vi "UI_page1.vi"(10 "传递队列输入":refnum<queue>, 11 "notifier":refnum<notifier>) -> ()   [LabVIEW 2012]
uses:
  <vilib>/GPower/VIRegister/Library/Convert/ToStr.vi
  <vilib>/GPower/VIRegister/Library/Convert/ToSGLArry.vi
  <vilib>/GPower/VIRegister/Library/Convert/ToI32.vi
  <vilib>/GPower/VIRegister/Library/SubVIs/FindRegisterData.vi
  <vilib>/GPower/VIRegister/Library/SubVIs/ReadSub.vi
  <vilib>/GPower/VIRegister/Library/SubVIs/WriteSub.vi
  <vilib>/GPower/VIRegister/Library/QManager/GetRegisterData.vi
  <vilib>/GPower/Error/Library/SetError.vi
  <vilib>/GPower/Error/Library/FilterCodes.vi
  <vilib>/GPower/Error/Library/Filter/FilterMulti.vi
  <vilib>/GPower/VIRegister/Library/QManager/QManagerAction.vi
  <vilib>/GPower/Error/Library/ErrorType.vi
  <vilib>/GPower/Error/Library/SplitAppended.vi
  <vilib>/GPower/Error/Library/SubVIs/ExplanationToError.vi
  <vilib>/GPower/VIRegister/Library/QManager/GetQName.vi
  <vilib>/GPower/VIRegister/Library/QManager/StartQManager.vi
  <vilib>/Utility/error.llb/Trim Whitespace.vi
  <vilib>/dlg_ctls.llb/Space Constant.vi
  <vilib>/Utility/error.llb/Error Code Database.vi
  <vilib>/GPower/Error/Library/SubVIs/SetStatus.vi
  <vilib>/GPower/Error/Library/AppendErrors.vi
  <vilib>/GPower/Error/Library/Append/AppendSingle.vi
  <vilib>/GPower/VIRegister/VIRegister.lvlib
  <vilib>/measure/NI_MABase.lvlib
panel:
  in  "选项卡控件":enum32{"光纤惯组数据设置", "主份1553B数据", "备份1553B数据"}(tab)
  in  "加表频率":dbl
  in  "加表幅值":dbl
  in  "陀螺频率":dbl
  in  "陀螺幅值":dbl
  in  "地检按钮":bool
  out "中断计数":i32
  out "模拟量显示区":string
  out "备份自检状态及船舱标志":string
  out "主份自检状态及船舱标志":string
  out "接收数据统计区域":string
  in  "备份加计3断电":bool
  in  "备份加计3加电":bool
  in  "备份陀螺3断电":bool
  in  "备份陀螺3加电":bool
  in  "备份温控关闭":bool
  in  "备份加计2断电":bool
  in  "备份加计1断电":bool
  in  "备份加计2加电":bool
  in  "备份加计1加电":bool
  in  "备份陀螺2断电":bool
  in  "备份陀螺1断电":bool
  in  "备份陀螺2加电":bool
  in  "备份陀螺1加电":bool
  in  "备份温控开启":bool
  in  "备份复位":bool
  in  "主份加计3断电":bool
  in  "主份加计3加电":bool
  in  "主份陀螺3断电":bool
  in  "主份陀螺3加电":bool
  in  "主份温控关闭":bool
  in  "主份加计2断电":bool
  in  "主份加计1断电":bool
  in  "主份加计2加电":bool
  in  "主份加计1加电":bool
  in  "主份陀螺2断电":bool
  in  "主份陀螺1断电":bool
  in  "主份陀螺2加电":bool
  in  "主份陀螺1加电":bool
  in  "主份温控开启":bool
  in  "主份复位":bool
  in  "备份复位远程终端":bool
  in  "备份取消发送器关闭":bool
  in  "备份发送器关闭":bool
  in  "备份发送上一状态字":bool
  in  "主份复位远程终端":bool
  in  "主份取消发送器关闭":bool
  in  "主份发送器关闭":bool
  in  "主份发送上一状态字":bool
  in  "备份RT地址选择":enum32{"RT31", "RT21", "RT9"}(radio)
  in  "主份RT地址选择":enum32{"RT31", "RT21", "RT9"}(radio)
  in  "备份通道选择":enum32{"通道A", "通道B"}(radio)
  in  "主份通道选择":enum32{"通道A", "通道B"}(radio)
  in  "备份自定义周期":dbl caption="ms"
  in  "备份周期设置":enum32{"160ms", "自定义", "480ms"}(radio)
  in  "主份自定义周期":dbl caption="ms"
  in  "主份周期设置":enum32{"160ms", "自定义", "480ms"}(radio)
  in  "设置存储信息":bool
  in  "备份存储":bool
  in  "主份存储":bool
  out "波形图表 12":dbl(graph)
  out "波形图表 11":dbl(graph)
  out "波形图表 10":dbl(graph)
  out "波形图表 9":dbl(graph)
  out "波形图表 8":dbl(graph)
  out "波形图表 7":dbl(graph)
  out "波形图表 6":dbl(graph)
  out "波形图表 5":dbl(graph)
  out "波形图表 4":dbl(graph)
  out "波形图表 3":dbl(graph)
  out "波形图表 2":dbl(graph)
  out "波形图表":dbl(graph)
  # "主份模式指令"
  # "测量存储区"
  # "备份模式指令"
  # "主份指令"
  # "备份指令"
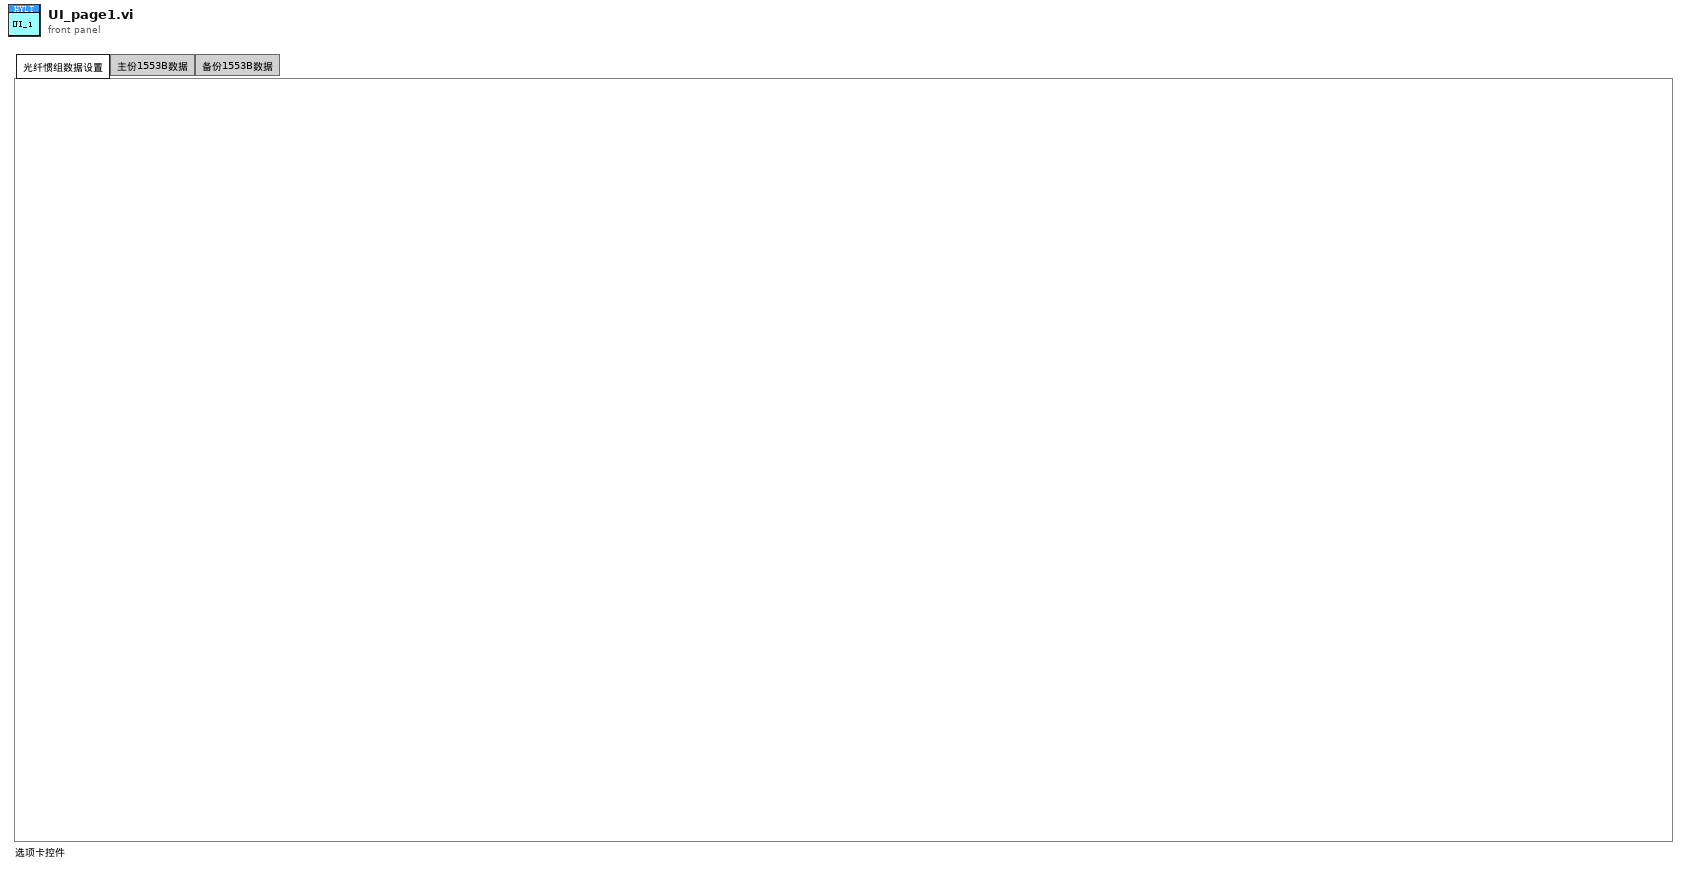
[diagram p1: front panel]
types:
  T1 = cluster{"主份通道选择":enum32{"通道A", "通道B"}, "备份通道选择":enum32{"通道A", "通道B"}}
  T2 = enum32{"invalid app kind", "Development System", "Run Time System", "Student Edition", "Embedded LabVIEW", "Evaluation", "Custom"}
  T3 = enum32{"Invalid", "Standard", "Closed", "Hidden", "Minimized", "Maximized"}
  T4 = cluster{"Core":cluster{"Current VI Reference":refnum<vi>, "Close Panel on Exit?":bool}, "传递队列输入":refnum<queue>, "信息帧":cluster{" 数据帧名称":string, " 数据":string, "备用操作符":bool, "起始地址":i32, "读写标志":i32, "长度":i32}, "主份控制指令":u16, "备份控制指令":u16}
  T5 = cluster{" 数据帧名称":string, " 数据":string, "备用操作符":bool, "起始地址":i32, "读写标志":i32, "长度":i32}
  T6 = cluster{"Current VI Reference":refnum<vi>, "Close Panel on Exit?":bool}
  T7 = cluster{"G1陀螺脉冲数":u32, "G2陀螺脉冲数":u32, "G3陀螺脉冲数":u32, "A1加速度计脉冲数":u32, "A2加速度计脉冲数":u32, "A3加速度计脉冲数":u32, "G1陀螺自检状态":u8, "G1陀螺光路温度":u8, "G2陀螺自检状态":u8, "G2陀螺光路温度":u8, "G3陀螺自检状态":u8, "G3陀螺光路温度":u8, "A1自检状态":u8, "A1幅值":u8, "A2自检状态":u8, "A2幅值":u8, "A3自检状态":u8, "A3幅值":u8, "IF1电路温度":u8, "IF2电路温度":u8, "IF3电路温度":u8, "温控自检字":u8, "加速度计温度测量字1":u32, "加速度计温度测量字2":u32, "LTU状态":u8, "帧计数":u8}
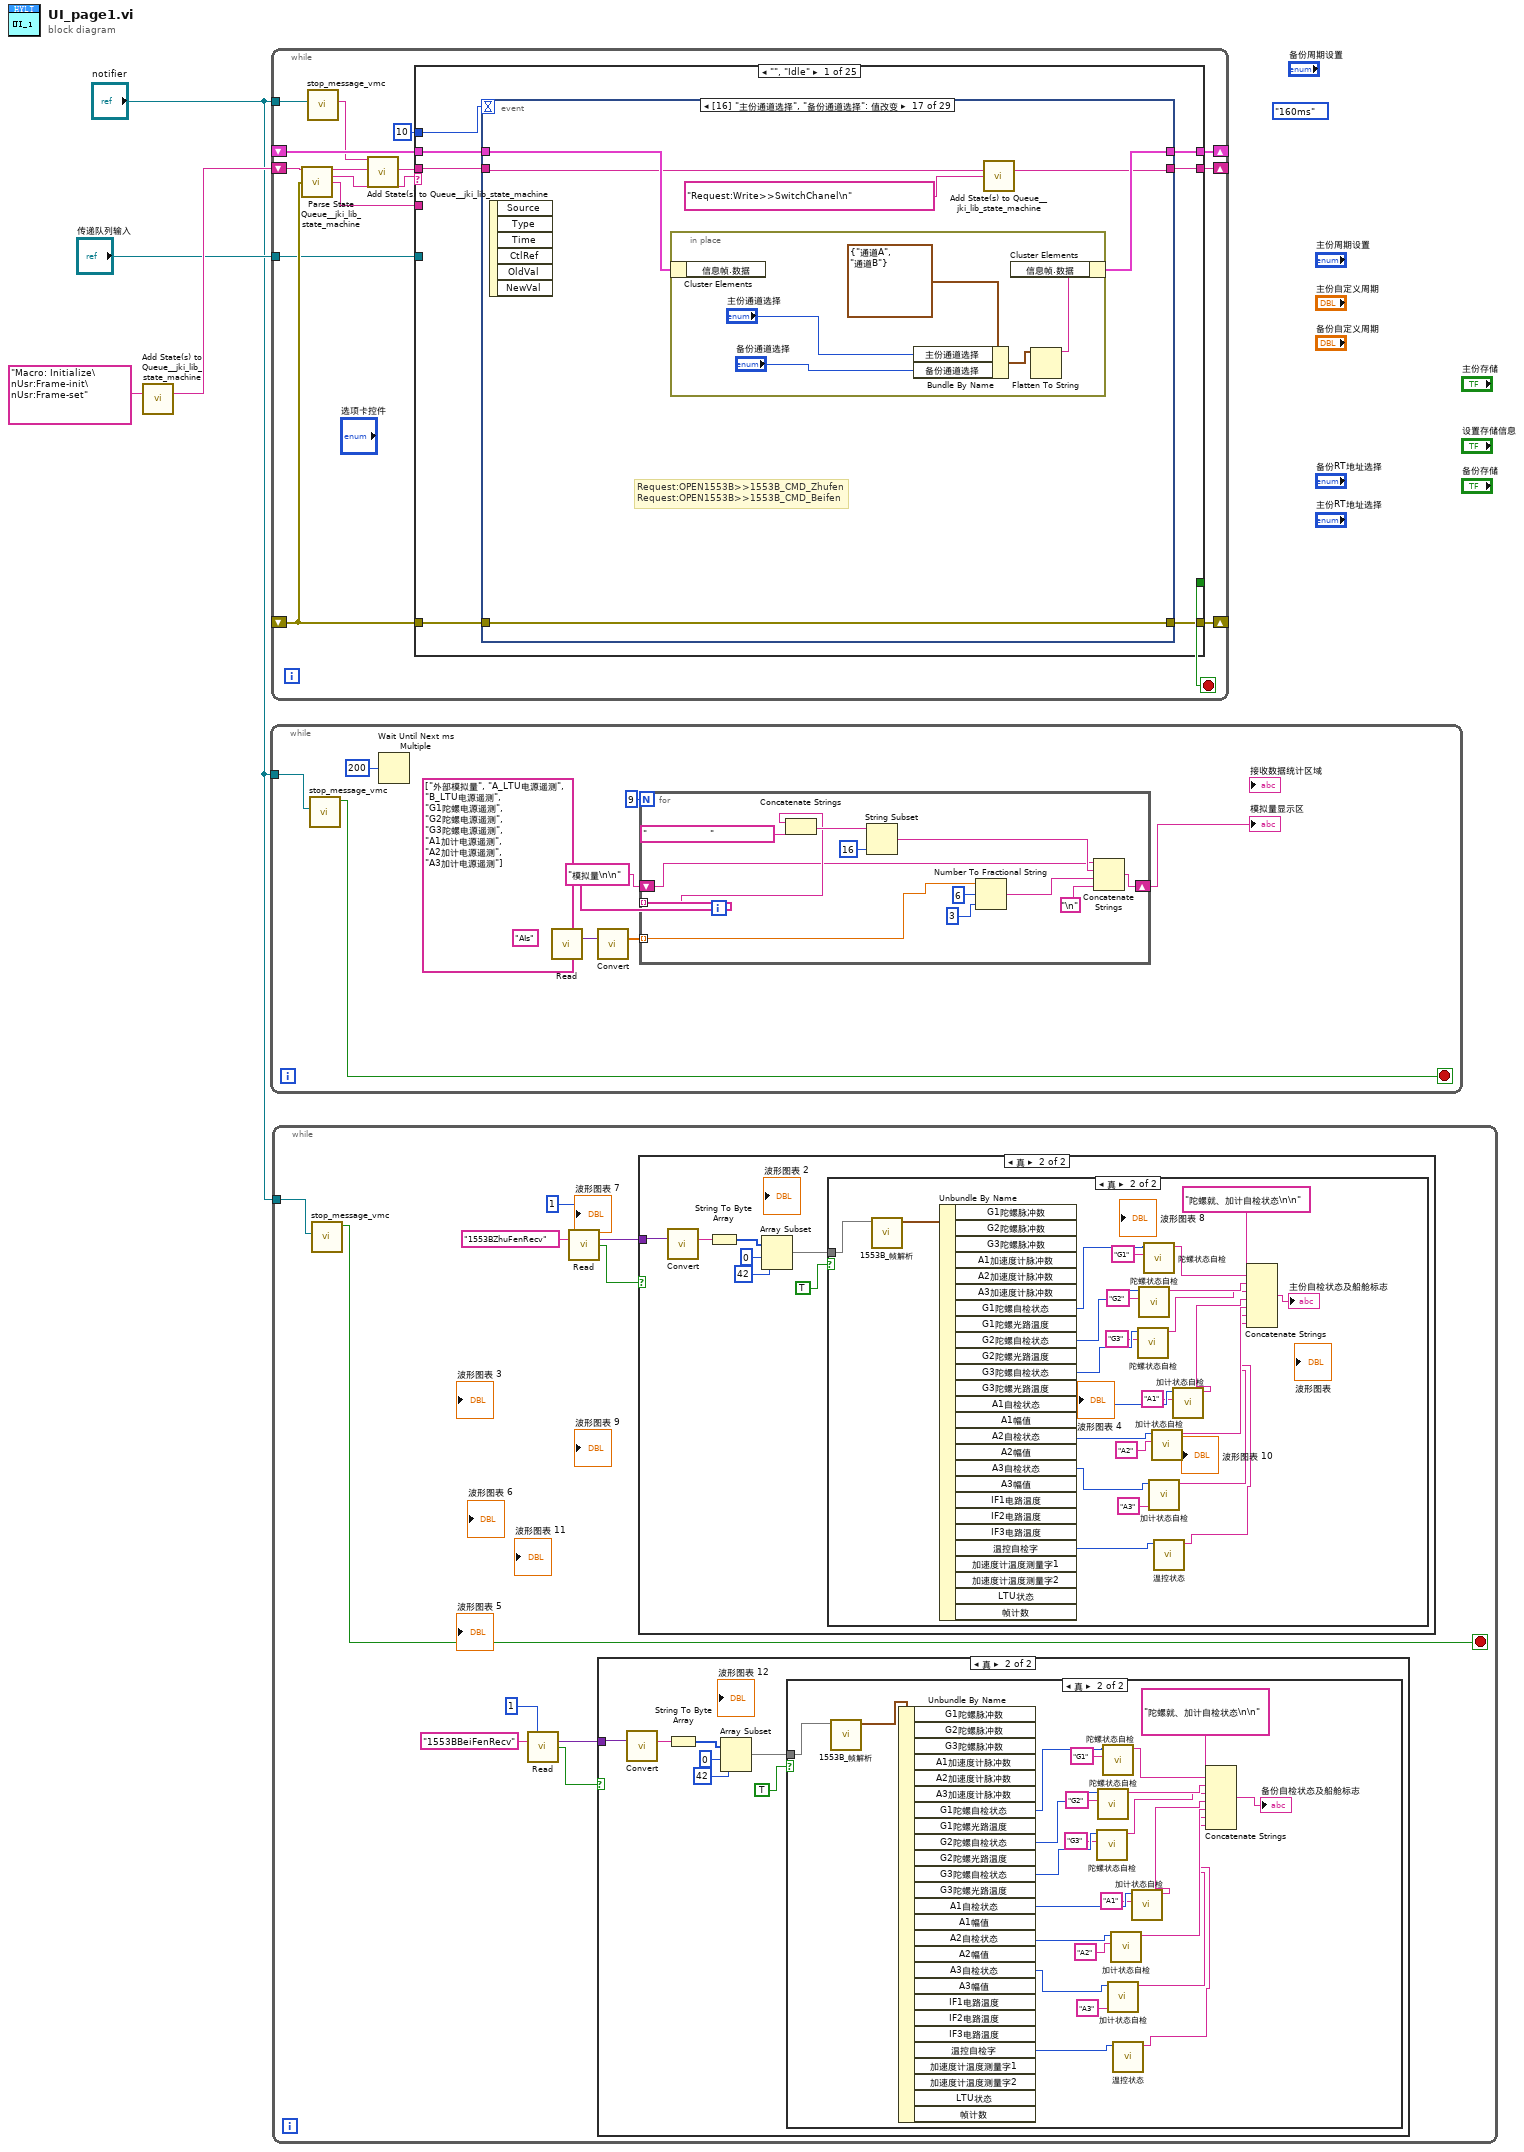
[diagram p0: block diagram]
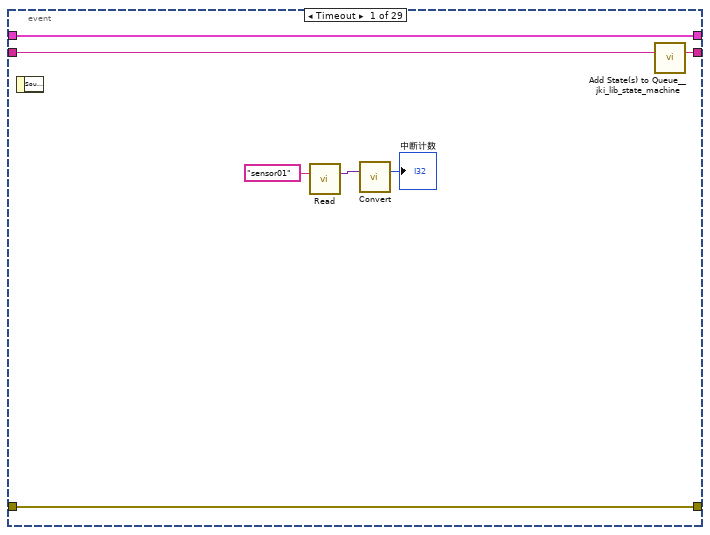
[diagram p6: hidden frame]
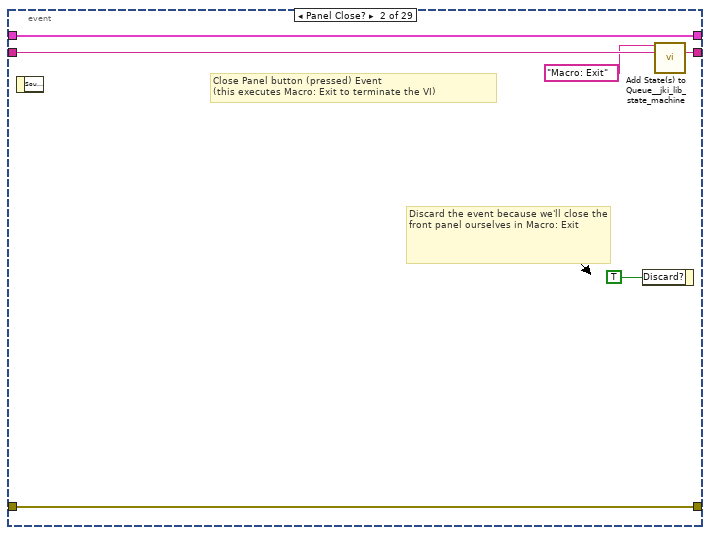
[diagram p7: hidden frame]
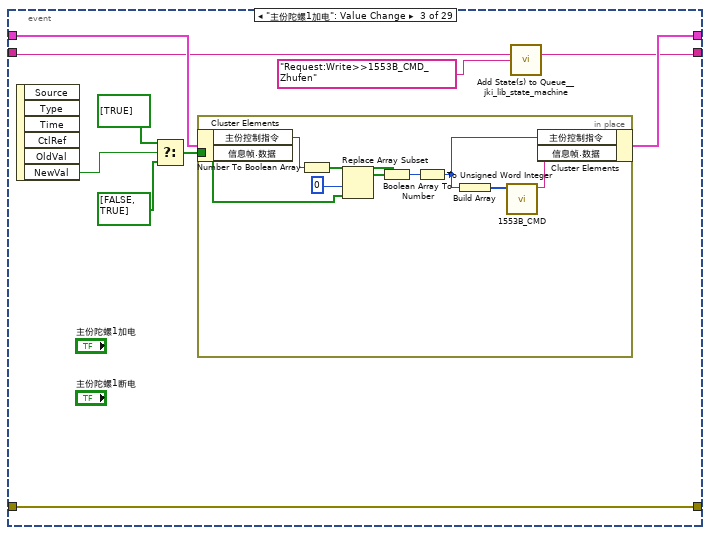
[diagram p8: hidden frame]
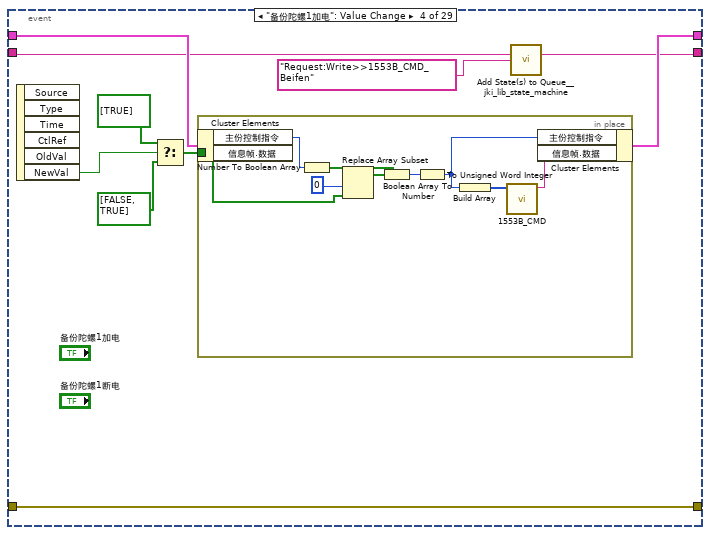
[diagram p9: hidden frame]
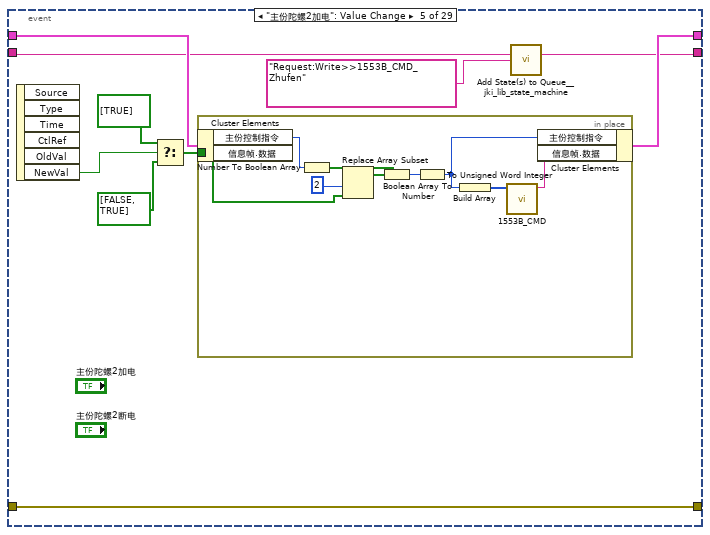
[diagram p10: hidden frame]
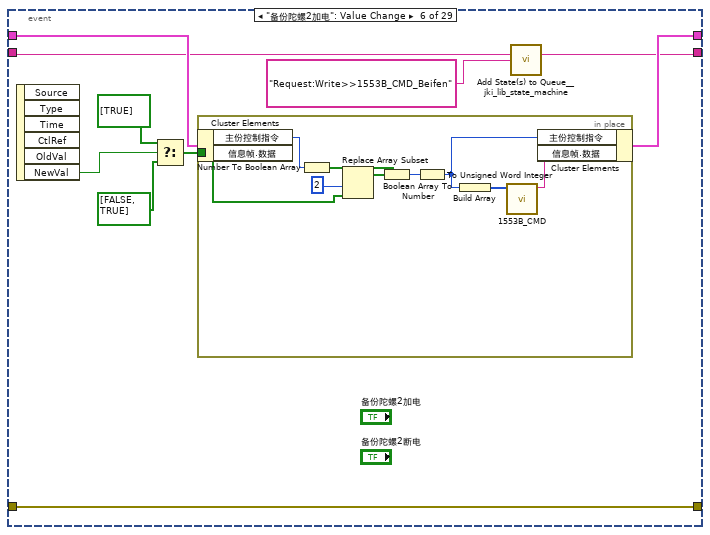
[diagram p11: hidden frame]
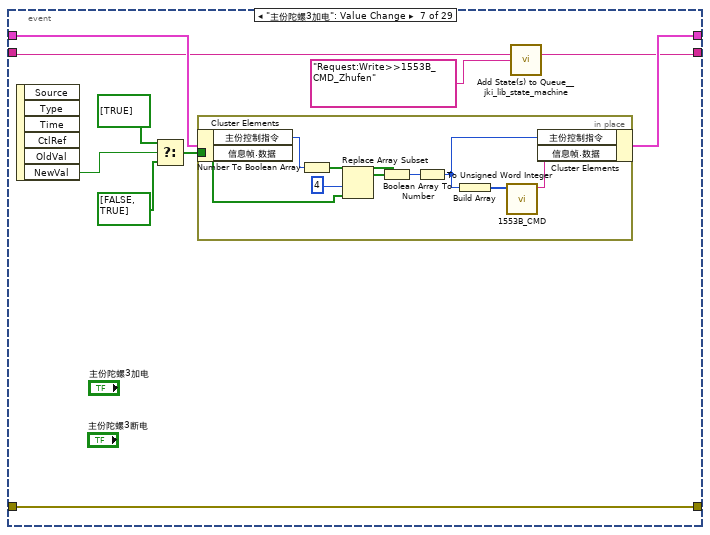
[diagram p12: hidden frame]
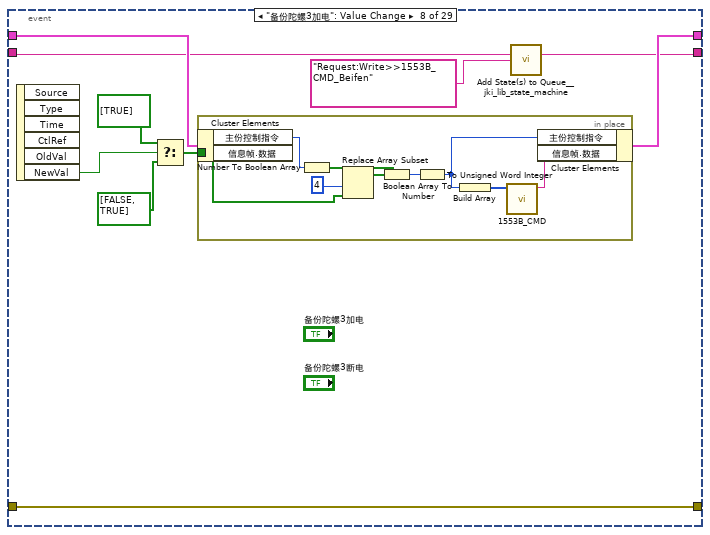
[diagram p13: hidden frame]
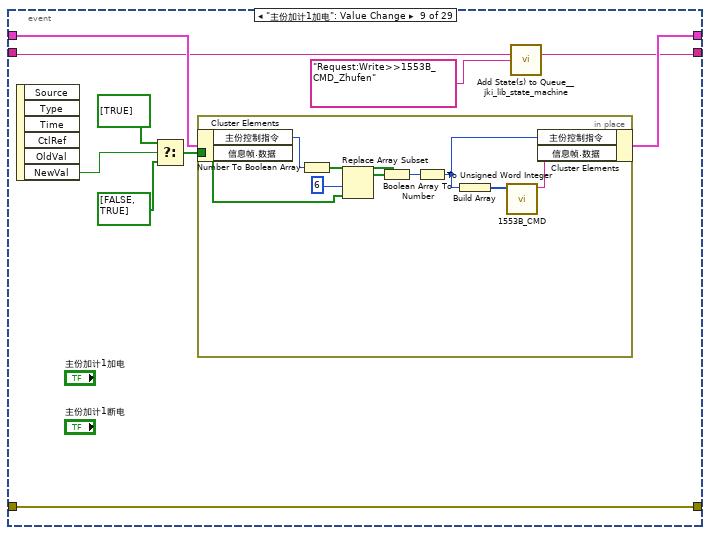
[diagram p14: hidden frame]
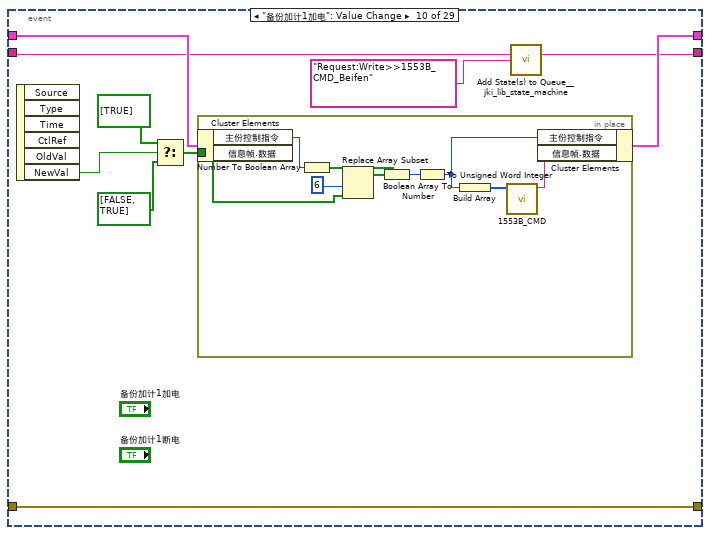
[diagram p15: hidden frame]
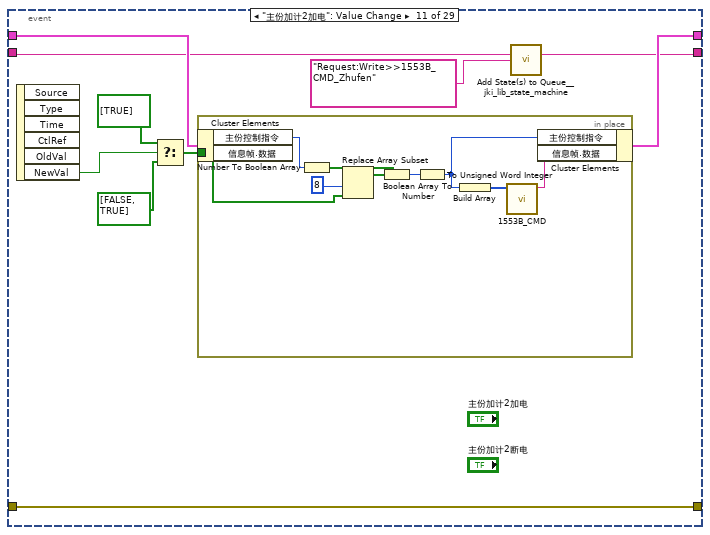
[diagram p16: hidden frame]
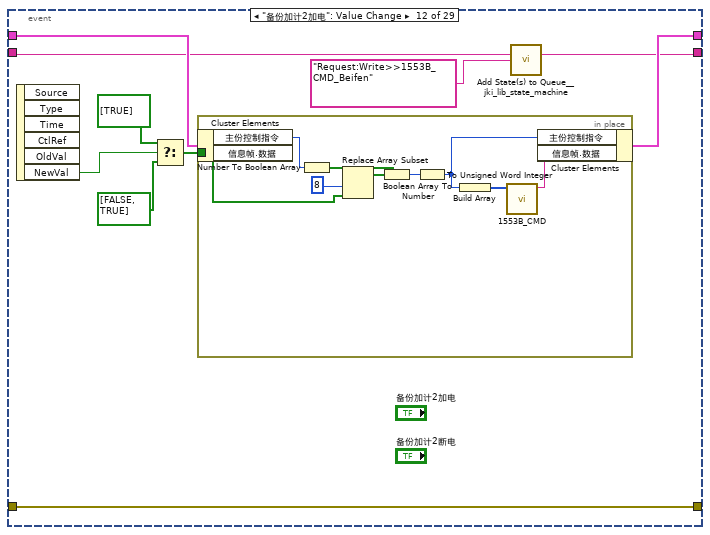
[diagram p17: hidden frame]
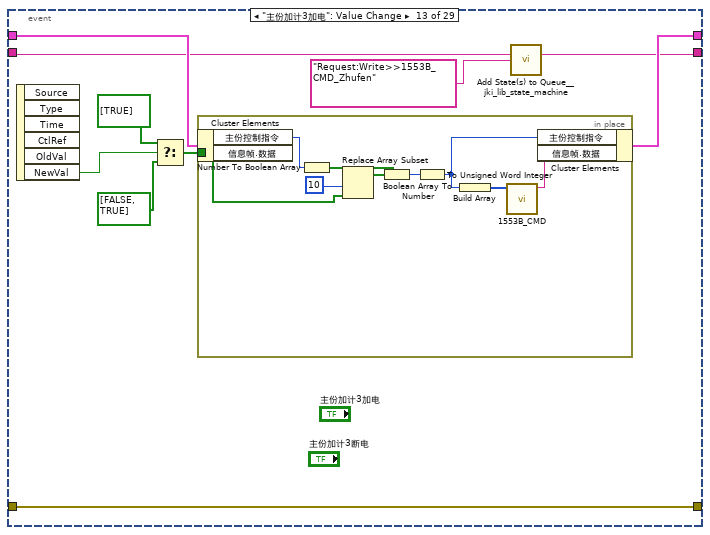
[diagram p18: hidden frame]
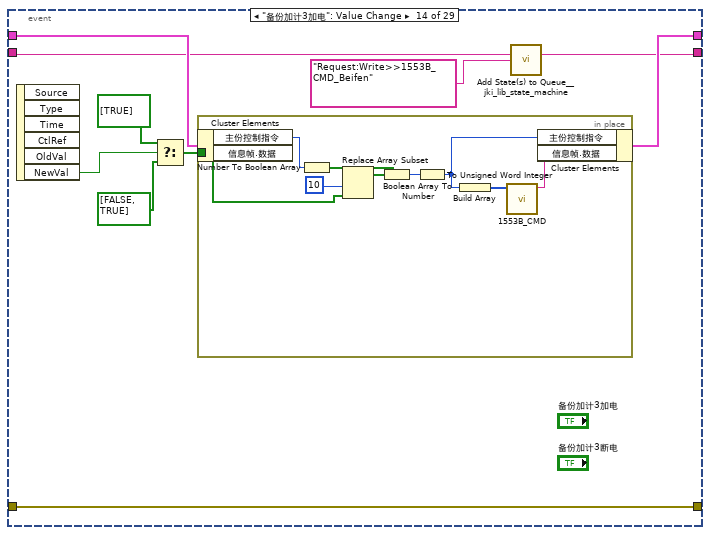
[diagram p19: hidden frame]
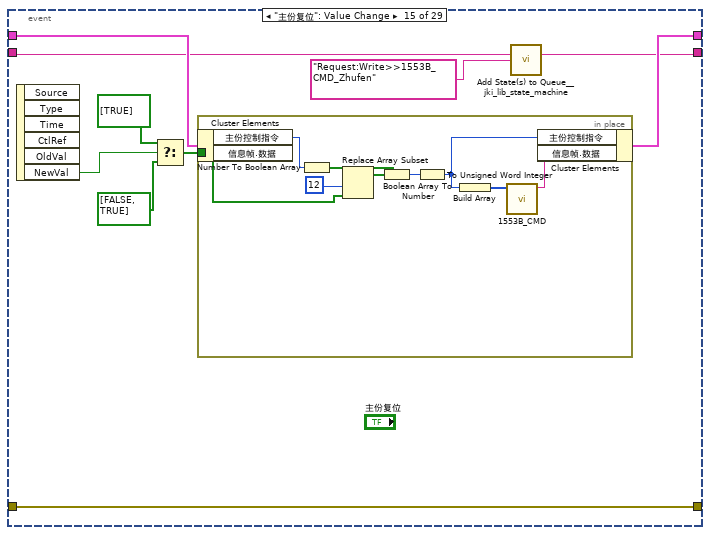
[diagram p20: hidden frame]
diagram:
  (unwired) enum32{"160ms", "自定义", "480ms"}."160ms" ("备份周期设置")
  n1 = call <vilib>:"Add State(s) to Queue__jki_lib_state_machine.vi"("State(s) in (\"\")"="Macro: Initialize\nUsr:Frame-init\nUsr:Frame-set") -> ("States Out"=w4:string)  [unwired: 14 in]
  n2 = while {
    tunnel: "notifier" -> [w13]
    stop <- w12 stop-if-true
    n3 = call "stop_message_vmc.vi"("notifier"=w13) -> ("Exit？"=w12:bool)  [unwired: 9 in, 1 out]
    n4 = Wait Until Next ms Multiple(millisecond multiple=u32 200 ("毫秒倍数")) -> ()  [unwired: 1 out]
    n5 = call <vilib>:"Read.vi"("Register name"="AIs") -> ("Register value"=w10:variant)  [unwired: 11 in, 3 out]
    n6 = call-poly <vilib>:"Convert.vi"("Register value in"=w10) -> ("Register value out"=w9:sgl[])  [unwired: 13 in, 1 out]
    n7 = for {
      N: 9 -> [_]
      tunnel: w9 -> [w21] mode=indexing
      shift-right: [w22] -> w7
      shift-left: "模拟量\n\n" -> [w15]
      tunnel: string[] ["外部模拟量", "A_LTU电源遥测", "B_LTU电源遥测", "G1陀螺电源遥测", "G2陀螺电源遥测", "G3陀螺电源遥测", "A1加计电源遥测", "A2加计电源遥测", "A3加计电源遥测"] -> [w16] mode=indexing
      n8 = Concatenate Strings(w16, "                     " ("字符串")) -> (w19:string)
      n9 = String Subset(string=w19, length (rest)=16 ("长度（剩余）")) -> (substring=w17:string)  [unwired: 1 in]
      n10 = Number To Fractional String(number=w21, width (-)=i16 6 ("宽度(-)"), precision (6)=i16 3 ("精度(6)")) -> (F-format string=w24:string)  [unwired: 1 in]
      n11 = Concatenate Strings(w15, w17, w24, "\n") -> (w22:string)
    }
    "模拟量显示区" <- w7
  }
  n12 = while "JKI - String-Based Queued State Machine (Basic) v1.0" {
    shift-right: [w35] -> _
    shift-left: _ -> [w34]
    shift-right: [w38] -> _
    shift-left: _ -> [w32]
    shift-right: [w37] -> _
    shift-left: w4 -> [w39]
    tunnel: "notifier" -> [w31]
    tunnel: "传递队列输入" -> [w27]
    stop <- w36 stop-if-true
    n13 = call <vilib>:"Parse State Queue__jki_lib_state_machine.vi"("State Queue"=w39, "Error In (no error)"=w32) -> ("Remaining States"=w30:string, "Current State"=w41:string, "Arguments"=w40:string)  [unwired: 11 in]
    n14 = call "stop_message_vmc.vi"("notifier"=w31) -> ("退出命令"=w29:string)  [unwired: 9 in, 1 out]
    n15 = call <vilib>:"Add State(s) to Queue__jki_lib_state_machine.vi"("State(s) in Front (\"\")"=w29, "State(s) in (\"\")"=w30) -> ("States Out"=w28:string)  [unwired: 13 in]
    n16 = case shown="\"\", \"Idle\"" w41 {
      selector: w41 -> [_ _ w490 _ _ _ _ _ _ _ _ _ _ _ _ _ _ _ _ _ _ _ _ _ _]
      tunnel: w28 -> [w42 w489 w494 w512 w518 w523 w527 w536 w542 w546 w550 w556 w566 w598 w603 w613 w617 w624 w644 w663 w689 w705 w710 w715 w727]
      tunnel: w40 -> [_ _ _ _ _ _ _ _ _ _ _ w551 w561 _ _ _ _ w618 w638 _ _ _ _ _ _]
      tunnel: w34 -> [w47 w486 w492 w503 w515 w521 w524 _ w537 w543 w548 w554 w562 w595 w600 w610 w614 w622 w642 w661 w687 w702 w707 w712 w723]
      tunnel: [w46 w487 w496 w509 errorcluster {"status"=FALSE, "code"=0, "source"=""} ("error out") w520 w525 w533 w538 w544 w547 w552 w563 w596 w601 w611 w615 w620 w640 w659 w685 w703 w708 w713 w725] -> w38
      tunnel: w32 -> [w45 w487 w495 w509 w514 w520 w525 w533 w539 w544 w547 w553 w564 w596 w601 w611 w615 w621 w641 w660 w686 w703 w708 w713 w725]
      tunnel: [w48 w488 w493 w511 w517 w522 w526 w535 w541 w545 w549 w555 w565 w597 w602 w612 w616 w623 w643 w662 w688 w704 w709 w714 w726] -> w37
      tunnel: [_ _ _ _ _ TRUE _ _ _ _ _ _ _ _ _ _ _ _ _ _ _ _ _ _ _] -> w36
      tunnel: [w44 w486 w492 w510 w515 w521 w524 w534 w537 w543 w548 w554 w562 w595 w600 w610 w614 w619 w639 w658 w684 w702 w707 w711 w723] -> w35
      tunnel: 10 ("Timeout") -> [w43 _ _ _ _ _ _ _ _ _ _ _ _ _ _ _ _ _ _ _ _ _ _ _ _]
      tunnel: w27 -> [_ _ _ _ _ _ _ w530 _ _ _ _ _ _ _ _ _ _ _ _ _ _ _ _ _]
      frame "", "Idle" {
        n17 = event shown="[16] \"主份通道选择\", \"备份通道选择\": 值改变" {
          selector: _ -> [_ _ _ _ _ _ _ _ _ _ _ _ _ _ _ _ _ _ _ _ _ _ _ _ _ _ _ _ _]
          dyn-events: _ -> [_ _ _ _ _ _ _ _ _ _ _ _ _ _ _ _ _ _ _ _ _ _ _ _ _ _ _ _ _]
          timeout: w43 -> [_ _ _ _ _ _ _ _ _ _ _ _ _ _ _ _ _ _ _ _ _ _ _ _ _ _ _ _ _]
          tunnel: w42 -> [w55 w61 w65 w84 w103 w122 w141 w160 w179 w198 w217 w236 w255 w274 w293 w312 w331 w342 w361 w380 w389 w398 w407 w416 w425 w434 w443 w455 w484]
          tunnel: [w54 w60 w63 w82 w101 w120 w139 w158 w177 w196 w215 w234 w253 w272 w291 w310 w329 w340 w359 w378 w387 w396 w405 w414 w423 w432 w441 w455 w484] -> w48
          tunnel: w47 -> [w52 w58 w71 w90 w109 w128 w147 w166 w185 w204 w223 w242 w261 w280 w299 w318 w333 w348 w367 w382 w391 w400 w409 w418 w427 w436 w445 w456 w485]
          tunnel: [w53 w59 w62 w81 w100 w119 w138 w157 w176 w195 w214 w233 w252 w271 w290 w309 w328 w339 w358 w377 w386 w395 w404 w413 w422 w431 w440 w454 w481] -> w46
          tunnel: w45 -> [w53 w59 w62 w81 w100 w119 w138 w157 w176 w195 w214 w233 w252 w271 w290 w309 w328 w339 w358 w377 w386 w395 w404 w413 w422 w431 w440 w454 w480]
          tunnel: [w52 w58 w66 w85 w104 w123 w142 w161 w180 w199 w218 w237 w256 w275 w294 w313 w332 w343 w362 w381 w390 w399 w408 w417 w426 w435 w444 w456 w485] -> w44
          event Timeout {
            n18 = event-data() -> ()  [unwired: 1 in, 1 out]
            n19 = call <vilib>:"Read.vi"("Register name"="sensor01") -> ("Register value"=w50:variant)  [unwired: 11 in, 3 out]
            n20 = call-poly <vilib>:"Convert.vi"("Register value in"=w50) -> ("Register value out"=→"中断计数":i32)  [unwired: 13 in, 1 out]
            n21 = call <vilib>:"Add State(s) to Queue__jki_lib_state_machine.vi"("State(s) in (\"\")"=w55) -> ("States Out"=w54:string)  [unwired: 14 in]
          }
          event Panel Close? {
            # "Discard the event because we'll close the front panel ourselves in Macro: Exit"
            # "Close Panel button (pressed) Event\n(this executes Macro: Exit to terminate the VI)"
            n22 = event-data() -> ()  [unwired: 1 in, 1 out]
            n23 = event-data("Discard?"=TRUE) -> ()  [unwired: 1 in, 1 out]
            n24 = call <vilib>:"Add State(s) to Queue__jki_lib_state_machine.vi"("State(s) in Front (\"\")"="Macro: Exit", "State(s) in (\"\")"=w61) -> ("States Out"=w60:string)  [unwired: 13 in]
          }
          event "主份陀螺1加电": Value Change {
            n25 = event-data() -> ("NewVal"=w70:bool)  [unwired: 1 in, 5 out]
            n26 = Select(t=bool[] [TRUE], s=w70, f=bool[] [FALSE, TRUE]) -> (s? t:f=w67:bool[])
            n27 = in-place {
              in-place-border: w67 -> [w75]
              n28 = in-place-cluster #1(w71) -> ("主份控制指令"=w80:u16)  [unwired: 1 out]
              n29 = Number To Boolean Array(number=w80) -> (Boolean array=w78:bool[])
              n30 = Replace Array Subset(array=w78, new element=w75, index=0 ("索引")) -> (w76:bool[])
              n31 = Boolean Array To Number(Boolean array=w76) -> (number=w79:u32)
              n32 = To Unsigned Word Integer(number=w79) -> (unsigned 16bit integer=w74:u16)
              n33 = Build Array(w74) -> (w73:u16[])
              n34 = call "1553B_CMD.vi"("数据字数组"=w73) -> ("1553B指令"=w72:string)  [unwired: 10 in]
              n35 = in-place-cluster #1("主份控制指令"=w74, "信息帧.数据"=w72) -> (w66:T4)
            }
            n36 = call <vilib>:"Add State(s) to Queue__jki_lib_state_machine.vi"("State(s) in (\"\")"=w65, "State(s) at Back (\"\")"="Request:Write>>1553B_CMD_Zhufen") -> ("States Out"=w63:string)  [unwired: 13 in]
          }
          event "备份陀螺1加电": Value Change {
            n37 = event-data() -> ("NewVal"=w89:bool)  [unwired: 1 in, 5 out]
            n38 = Select(t=bool[] [TRUE], s=w89, f=bool[] [FALSE, TRUE]) -> (s? t:f=w86:bool[])
            n39 = in-place {
              in-place-border: w86 -> [w94]
              n40 = in-place-cluster #2(w90) -> ("主份控制指令"=w99:u16)  [unwired: 1 out]
              n41 = Number To Boolean Array(number=w99) -> (Boolean array=w97:bool[])
              n42 = Replace Array Subset(array=w97, new element=w94, index=0 ("索引")) -> (w95:bool[])
              n43 = Boolean Array To Number(Boolean array=w95) -> (number=w98:u32)
              n44 = To Unsigned Word Integer(number=w98) -> (unsigned 16bit integer=w93:u16)
              n45 = Build Array(w93) -> (w92:u16[])
              n46 = call "1553B_CMD.vi"("数据字数组"=w92) -> ("1553B指令"=w91:string)  [unwired: 10 in]
              n47 = in-place-cluster #2("主份控制指令"=w93, "信息帧.数据"=w91) -> (w85:T4)
            }
            n48 = call <vilib>:"Add State(s) to Queue__jki_lib_state_machine.vi"("State(s) in (\"\")"=w84, "State(s) at Back (\"\")"="Request:Write>>1553B_CMD_Beifen") -> ("States Out"=w82:string)  [unwired: 13 in]
          }
          event "主份陀螺2加电": Value Change {
            n49 = event-data() -> ("NewVal"=w108:bool)  [unwired: 1 in, 5 out]
            n50 = Select(t=bool[] [TRUE], s=w108, f=bool[] [FALSE, TRUE]) -> (s? t:f=w105:bool[])
            n51 = in-place {
              in-place-border: w105 -> [w113]
              n52 = in-place-cluster #3(w109) -> ("主份控制指令"=w118:u16)  [unwired: 1 out]
              n53 = Number To Boolean Array(number=w118) -> (Boolean array=w116:bool[])
              n54 = Replace Array Subset(array=w116, new element=w113, index=2 ("索引")) -> (w114:bool[])
              n55 = Boolean Array To Number(Boolean array=w114) -> (number=w117:u32)
              n56 = To Unsigned Word Integer(number=w117) -> (unsigned 16bit integer=w112:u16)
              n57 = Build Array(w112) -> (w111:u16[])
              n58 = call "1553B_CMD.vi"("数据字数组"=w111) -> ("1553B指令"=w110:string)  [unwired: 10 in]
              n59 = in-place-cluster #3("主份控制指令"=w112, "信息帧.数据"=w110) -> (w104:T4)
            }
            n60 = call <vilib>:"Add State(s) to Queue__jki_lib_state_machine.vi"("State(s) in (\"\")"=w103, "State(s) at Back (\"\")"="Request:Write>>1553B_CMD_Zhufen") -> ("States Out"=w101:string)  [unwired: 13 in]
          }
          event "备份陀螺2加电": Value Change {
            n61 = event-data() -> ("NewVal"=w127:bool)  [unwired: 1 in, 5 out]
            n62 = Select(t=bool[] [TRUE], s=w127, f=bool[] [FALSE, TRUE]) -> (s? t:f=w124:bool[])
            n63 = in-place {
              in-place-border: w124 -> [w132]
              n64 = in-place-cluster #4(w128) -> ("主份控制指令"=w137:u16)  [unwired: 1 out]
              n65 = Number To Boolean Array(number=w137) -> (Boolean array=w135:bool[])
              n66 = Replace Array Subset(array=w135, new element=w132, index=2 ("索引")) -> (w133:bool[])
              n67 = Boolean Array To Number(Boolean array=w133) -> (number=w136:u32)
              n68 = To Unsigned Word Integer(number=w136) -> (unsigned 16bit integer=w131:u16)
              n69 = Build Array(w131) -> (w130:u16[])
              n70 = call "1553B_CMD.vi"("数据字数组"=w130) -> ("1553B指令"=w129:string)  [unwired: 10 in]
              n71 = in-place-cluster #4("主份控制指令"=w131, "信息帧.数据"=w129) -> (w123:T4)
            }
            n72 = call <vilib>:"Add State(s) to Queue__jki_lib_state_machine.vi"("State(s) in (\"\")"=w122, "State(s) at Back (\"\")"="Request:Write>>1553B_CMD_Beifen") -> ("States Out"=w120:string)  [unwired: 13 in]
          }
          event "主份陀螺3加电": Value Change {
            n73 = event-data() -> ("NewVal"=w146:bool)  [unwired: 1 in, 5 out]
            n74 = Select(t=bool[] [TRUE], s=w146, f=bool[] [FALSE, TRUE]) -> (s? t:f=w143:bool[])
            n75 = in-place {
              in-place-border: w143 -> [w151]
              n76 = in-place-cluster #5(w147) -> ("主份控制指令"=w156:u16)  [unwired: 1 out]
              n77 = Number To Boolean Array(number=w156) -> (Boolean array=w154:bool[])
              n78 = Replace Array Subset(array=w154, new element=w151, index=4 ("索引")) -> (w152:bool[])
              n79 = Boolean Array To Number(Boolean array=w152) -> (number=w155:u32)
              n80 = To Unsigned Word Integer(number=w155) -> (unsigned 16bit integer=w150:u16)
              n81 = Build Array(w150) -> (w149:u16[])
              n82 = call "1553B_CMD.vi"("数据字数组"=w149) -> ("1553B指令"=w148:string)  [unwired: 10 in]
              n83 = in-place-cluster #5("主份控制指令"=w150, "信息帧.数据"=w148) -> (w142:T4)
            }
            n84 = call <vilib>:"Add State(s) to Queue__jki_lib_state_machine.vi"("State(s) in (\"\")"=w141, "State(s) at Back (\"\")"="Request:Write>>1553B_CMD_Zhufen") -> ("States Out"=w139:string)  [unwired: 13 in]
          }
          event "备份陀螺3加电": Value Change {
            n85 = event-data() -> ("NewVal"=w165:bool)  [unwired: 1 in, 5 out]
            n86 = Select(t=bool[] [TRUE], s=w165, f=bool[] [FALSE, TRUE]) -> (s? t:f=w162:bool[])
            n87 = in-place {
              in-place-border: w162 -> [w170]
              n88 = in-place-cluster #6(w166) -> ("主份控制指令"=w175:u16)  [unwired: 1 out]
              n89 = Number To Boolean Array(number=w175) -> (Boolean array=w173:bool[])
              n90 = Replace Array Subset(array=w173, new element=w170, index=4 ("索引")) -> (w171:bool[])
              n91 = Boolean Array To Number(Boolean array=w171) -> (number=w174:u32)
              n92 = To Unsigned Word Integer(number=w174) -> (unsigned 16bit integer=w169:u16)
              n93 = Build Array(w169) -> (w168:u16[])
              n94 = call "1553B_CMD.vi"("数据字数组"=w168) -> ("1553B指令"=w167:string)  [unwired: 10 in]
              n95 = in-place-cluster #6("主份控制指令"=w169, "信息帧.数据"=w167) -> (w161:T4)
            }
            n96 = call <vilib>:"Add State(s) to Queue__jki_lib_state_machine.vi"("State(s) in (\"\")"=w160, "State(s) at Back (\"\")"="Request:Write>>1553B_CMD_Beifen") -> ("States Out"=w158:string)  [unwired: 13 in]
          }
          event "主份加计1加电": Value Change {
            n97 = event-data() -> ("NewVal"=w184:bool)  [unwired: 1 in, 5 out]
            n98 = Select(t=bool[] [TRUE], s=w184, f=bool[] [FALSE, TRUE]) -> (s? t:f=w181:bool[])
            n99 = in-place {
              in-place-border: w181 -> [w189]
              n100 = in-place-cluster #7(w185) -> ("主份控制指令"=w194:u16)  [unwired: 1 out]
              n101 = Number To Boolean Array(number=w194) -> (Boolean array=w192:bool[])
              n102 = Replace Array Subset(array=w192, new element=w189, index=6 ("索引")) -> (w190:bool[])
              n103 = Boolean Array To Number(Boolean array=w190) -> (number=w193:u32)
              n104 = To Unsigned Word Integer(number=w193) -> (unsigned 16bit integer=w188:u16)
              n105 = Build Array(w188) -> (w187:u16[])
              n106 = call "1553B_CMD.vi"("数据字数组"=w187) -> ("1553B指令"=w186:string)  [unwired: 10 in]
              n107 = in-place-cluster #7("主份控制指令"=w188, "信息帧.数据"=w186) -> (w180:T4)
            }
            n108 = call <vilib>:"Add State(s) to Queue__jki_lib_state_machine.vi"("State(s) in (\"\")"=w179, "State(s) at Back (\"\")"="Request:Write>>1553B_CMD_Zhufen") -> ("States Out"=w177:string)  [unwired: 13 in]
          }
          event "备份加计1加电": Value Change {
            n109 = event-data() -> ("NewVal"=w203:bool)  [unwired: 1 in, 5 out]
            n110 = Select(t=bool[] [TRUE], s=w203, f=bool[] [FALSE, TRUE]) -> (s? t:f=w200:bool[])
            n111 = in-place {
              in-place-border: w200 -> [w208]
              n112 = in-place-cluster #8(w204) -> ("主份控制指令"=w213:u16)  [unwired: 1 out]
              n113 = Number To Boolean Array(number=w213) -> (Boolean array=w211:bool[])
              n114 = Replace Array Subset(array=w211, new element=w208, index=6 ("索引")) -> (w209:bool[])
              n115 = Boolean Array To Number(Boolean array=w209) -> (number=w212:u32)
              n116 = To Unsigned Word Integer(number=w212) -> (unsigned 16bit integer=w207:u16)
              n117 = Build Array(w207) -> (w206:u16[])
              n118 = call "1553B_CMD.vi"("数据字数组"=w206) -> ("1553B指令"=w205:string)  [unwired: 10 in]
              n119 = in-place-cluster #8("主份控制指令"=w207, "信息帧.数据"=w205) -> (w199:T4)
            }
            n120 = call <vilib>:"Add State(s) to Queue__jki_lib_state_machine.vi"("State(s) in (\"\")"=w198, "State(s) at Back (\"\")"="Request:Write>>1553B_CMD_Beifen") -> ("States Out"=w196:string)  [unwired: 13 in]
          }
          event "主份加计2加电": Value Change {
            n121 = event-data() -> ("NewVal"=w222:bool)  [unwired: 1 in, 5 out]
            n122 = Select(t=bool[] [TRUE], s=w222, f=bool[] [FALSE, TRUE]) -> (s? t:f=w219:bool[])
            n123 = in-place {
              in-place-border: w219 -> [w227]
              n124 = in-place-cluster #9(w223) -> ("主份控制指令"=w232:u16)  [unwired: 1 out]
              n125 = Number To Boolean Array(number=w232) -> (Boolean array=w230:bool[])
              n126 = Replace Array Subset(array=w230, new element=w227, index=8 ("索引")) -> (w228:bool[])
              n127 = Boolean Array To Number(Boolean array=w228) -> (number=w231:u32)
              n128 = To Unsigned Word Integer(number=w231) -> (unsigned 16bit integer=w226:u16)
              n129 = Build Array(w226) -> (w225:u16[])
              n130 = call "1553B_CMD.vi"("数据字数组"=w225) -> ("1553B指令"=w224:string)  [unwired: 10 in]
              n131 = in-place-cluster #9("主份控制指令"=w226, "信息帧.数据"=w224) -> (w218:T4)
            }
            n132 = call <vilib>:"Add State(s) to Queue__jki_lib_state_machine.vi"("State(s) in (\"\")"=w217, "State(s) at Back (\"\")"="Request:Write>>1553B_CMD_Zhufen") -> ("States Out"=w215:string)  [unwired: 13 in]
          }
          event "备份加计2加电": Value Change {
            n133 = event-data() -> ("NewVal"=w241:bool)  [unwired: 1 in, 5 out]
            n134 = Select(t=bool[] [TRUE], s=w241, f=bool[] [FALSE, TRUE]) -> (s? t:f=w238:bool[])
            n135 = in-place {
              in-place-border: w238 -> [w246]
              n136 = in-place-cluster #10(w242) -> ("主份控制指令"=w251:u16)  [unwired: 1 out]
              n137 = Number To Boolean Array(number=w251) -> (Boolean array=w249:bool[])
              n138 = Replace Array Subset(array=w249, new element=w246, index=8 ("索引")) -> (w247:bool[])
              n139 = Boolean Array To Number(Boolean array=w247) -> (number=w250:u32)
              n140 = To Unsigned Word Integer(number=w250) -> (unsigned 16bit integer=w245:u16)
              n141 = Build Array(w245) -> (w244:u16[])
              n142 = call "1553B_CMD.vi"("数据字数组"=w244) -> ("1553B指令"=w243:string)  [unwired: 10 in]
              n143 = in-place-cluster #10("主份控制指令"=w245, "信息帧.数据"=w243) -> (w237:T4)
            }
            n144 = call <vilib>:"Add State(s) to Queue__jki_lib_state_machine.vi"("State(s) in (\"\")"=w236, "State(s) at Back (\"\")"="Request:Write>>1553B_CMD_Beifen") -> ("States Out"=w234:string)  [unwired: 13 in]
          }
          event "主份加计3加电": Value Change {
            n145 = event-data() -> ("NewVal"=w260:bool)  [unwired: 1 in, 5 out]
            n146 = Select(t=bool[] [TRUE], s=w260, f=bool[] [FALSE, TRUE]) -> (s? t:f=w257:bool[])
            n147 = in-place {
              in-place-border: w257 -> [w265]
              n148 = in-place-cluster #11(w261) -> ("主份控制指令"=w270:u16)  [unwired: 1 out]
              n149 = Number To Boolean Array(number=w270) -> (Boolean array=w268:bool[])
              n150 = Replace Array Subset(array=w268, new element=w265, index=10 ("索引")) -> (w266:bool[])
              n151 = Boolean Array To Number(Boolean array=w266) -> (number=w269:u32)
              n152 = To Unsigned Word Integer(number=w269) -> (unsigned 16bit integer=w264:u16)
              n153 = Build Array(w264) -> (w263:u16[])
              n154 = call "1553B_CMD.vi"("数据字数组"=w263) -> ("1553B指令"=w262:string)  [unwired: 10 in]
              n155 = in-place-cluster #11("主份控制指令"=w264, "信息帧.数据"=w262) -> (w256:T4)
            }
            n156 = call <vilib>:"Add State(s) to Queue__jki_lib_state_machine.vi"("State(s) in (\"\")"=w255, "State(s) at Back (\"\")"="Request:Write>>1553B_CMD_Zhufen") -> ("States Out"=w253:string)  [unwired: 13 in]
          }
          event "备份加计3加电": Value Change {
            n157 = event-data() -> ("NewVal"=w279:bool)  [unwired: 1 in, 5 out]
            n158 = Select(t=bool[] [TRUE], s=w279, f=bool[] [FALSE, TRUE]) -> (s? t:f=w276:bool[])
            n159 = in-place {
              in-place-border: w276 -> [w284]
              n160 = in-place-cluster #12(w280) -> ("主份控制指令"=w289:u16)  [unwired: 1 out]
              n161 = Number To Boolean Array(number=w289) -> (Boolean array=w287:bool[])
              n162 = Replace Array Subset(array=w287, new element=w284, index=10 ("索引")) -> (w285:bool[])
              n163 = Boolean Array To Number(Boolean array=w285) -> (number=w288:u32)
              n164 = To Unsigned Word Integer(number=w288) -> (unsigned 16bit integer=w283:u16)
              n165 = Build Array(w283) -> (w282:u16[])
              n166 = call "1553B_CMD.vi"("数据字数组"=w282) -> ("1553B指令"=w281:string)  [unwired: 10 in]
              n167 = in-place-cluster #12("主份控制指令"=w283, "信息帧.数据"=w281) -> (w275:T4)
            }
            n168 = call <vilib>:"Add State(s) to Queue__jki_lib_state_machine.vi"("State(s) in (\"\")"=w274, "State(s) at Back (\"\")"="Request:Write>>1553B_CMD_Beifen") -> ("States Out"=w272:string)  [unwired: 13 in]
          }
          event "主份复位": Value Change {
            n169 = event-data() -> ("NewVal"=w298:bool)  [unwired: 1 in, 5 out]
            n170 = Select(t=bool[] [TRUE], s=w298, f=bool[] [FALSE, TRUE]) -> (s? t:f=w295:bool[])
            n171 = in-place {
              in-place-border: w295 -> [w303]
              n172 = in-place-cluster #13(w299) -> ("主份控制指令"=w308:u16)  [unwired: 1 out]
              n173 = Number To Boolean Array(number=w308) -> (Boolean array=w306:bool[])
              n174 = Replace Array Subset(array=w306, new element=w303, index=12 ("索引")) -> (w304:bool[])
              n175 = Boolean Array To Number(Boolean array=w304) -> (number=w307:u32)
              n176 = To Unsigned Word Integer(number=w307) -> (unsigned 16bit integer=w302:u16)
              n177 = Build Array(w302) -> (w301:u16[])
              n178 = call "1553B_CMD.vi"("数据字数组"=w301) -> ("1553B指令"=w300:string)  [unwired: 10 in]
              n179 = in-place-cluster #13("主份控制指令"=w302, "信息帧.数据"=w300) -> (w294:T4)
            }
            n180 = call <vilib>:"Add State(s) to Queue__jki_lib_state_machine.vi"("State(s) in (\"\")"=w293, "State(s) at Back (\"\")"="Request:Write>>1553B_CMD_Zhufen") -> ("States Out"=w291:string)  [unwired: 13 in]
          }
          event "备份复位": Value Change {
            n181 = event-data() -> ("NewVal"=w317:bool)  [unwired: 1 in, 5 out]
            n182 = Select(t=bool[] [TRUE], s=w317, f=bool[] [FALSE, TRUE]) -> (s? t:f=w314:bool[])
            n183 = in-place {
              in-place-border: w314 -> [w322]
              n184 = in-place-cluster #14(w318) -> ("主份控制指令"=w327:u16)  [unwired: 1 out]
              n185 = Number To Boolean Array(number=w327) -> (Boolean array=w325:bool[])
              n186 = Replace Array Subset(array=w325, new element=w322, index=12 ("索引")) -> (w323:bool[])
              n187 = Boolean Array To Number(Boolean array=w323) -> (number=w326:u32)
              n188 = To Unsigned Word Integer(number=w326) -> (unsigned 16bit integer=w321:u16)
              n189 = Build Array(w321) -> (w320:u16[])
              n190 = call "1553B_CMD.vi"("数据字数组"=w320) -> ("1553B指令"=w319:string)  [unwired: 10 in]
              n191 = in-place-cluster #14("主份控制指令"=w321, "信息帧.数据"=w319) -> (w313:T4)
            }
            n192 = call <vilib>:"Add State(s) to Queue__jki_lib_state_machine.vi"("State(s) in (\"\")"=w312, "State(s) at Back (\"\")"="Request:Write>>1553B_CMD_Beifen") -> ("States Out"=w310:string)  [unwired: 13 in]
          }
          event "主份通道选择", "备份通道选择": Value Change {
            # "Request:OPEN1553B>>1553B_CMD_Zhufen\nRequest:OPEN1553B>>1553B_CMD_Beifen"
            n193 = event-data() -> ()  [unwired: 1 in, 6 out]
            n194 = in-place {
              n195 = in-place-cluster #15(w333) -> ()  [unwired: 1 out]
              n196 = Bundle By Name(cluster=T1 {"主份通道选择"=enum."通道A", "备份通道选择"=enum."通道B"} ("输入簇"), "主份通道选择"="主份通道选择", "备份通道选择"="备份通道选择") -> (w335:T1)
              n197 = Flatten To String(anything=w335) -> (data string=w334:string)  [unwired: 3 in, 2 out]
              n198 = in-place-cluster #15("信息帧.数据"=w334) -> (w332:T4)
            }
            n199 = call <vilib>:"Add State(s) to Queue__jki_lib_state_machine.vi"("State(s) in (\"\")"=w331, "State(s) at Back (\"\")"="Request:Write>>SwitchChanel\n") -> ("States Out"=w329:string)  [unwired: 13 in]
          }
          event "主份温控开启": Value Change {
            n200 = event-data() -> ("NewVal"=w347:bool)  [unwired: 1 in, 5 out]
            n201 = Select(t=bool[] [TRUE, FALSE], s=w347, f=bool[] [FALSE, TRUE]) -> (s? t:f=w344:bool[])
            n202 = in-place {
              in-place-border: w344 -> [w352]
              n203 = in-place-cluster #16(w348) -> ("主份控制指令"=w357:u16)  [unwired: 1 out]
              n204 = Number To Boolean Array(number=w357) -> (Boolean array=w355:bool[])
              n205 = Replace Array Subset(array=w355, new element=w352, index=14 ("索引")) -> (w353:bool[])
              n206 = Boolean Array To Number(Boolean array=w353) -> (number=w356:u32)
              n207 = To Unsigned Word Integer(number=w356) -> (unsigned 16bit integer=w351:u16)
              n208 = Build Array(w351) -> (w350:u16[])
              n209 = call "1553B_CMD.vi"("数据字数组"=w350) -> ("1553B指令"=w349:string)  [unwired: 10 in]
              n210 = in-place-cluster #16("主份控制指令"=w351, "信息帧.数据"=w349) -> (w343:T4)
            }
            n211 = call <vilib>:"Add State(s) to Queue__jki_lib_state_machine.vi"("State(s) in (\"\")"=w342, "State(s) at Back (\"\")"="Request:Write>>1553B_CMD_Zhufen") -> ("States Out"=w340:string)  [unwired: 13 in]
          }
          event "备份温控开启": Value Change {
            n212 = event-data() -> ("NewVal"=w366:bool)  [unwired: 1 in, 5 out]
            n213 = Select(t=bool[] [TRUE, FALSE], s=w366, f=bool[] [FALSE, TRUE]) -> (s? t:f=w363:bool[])
            n214 = in-place {
              in-place-border: w363 -> [w371]
              n215 = in-place-cluster #17(w367) -> ("主份控制指令"=w376:u16)  [unwired: 1 out]
              n216 = Number To Boolean Array(number=w376) -> (Boolean array=w374:bool[])
              n217 = Replace Array Subset(array=w374, new element=w371, index=14 ("索引")) -> (w372:bool[])
              n218 = Boolean Array To Number(Boolean array=w372) -> (number=w375:u32)
              n219 = To Unsigned Word Integer(number=w375) -> (unsigned 16bit integer=w370:u16)
              n220 = Build Array(w370) -> (w369:u16[])
              n221 = call "1553B_CMD.vi"("数据字数组"=w369) -> ("1553B指令"=w368:string)  [unwired: 10 in]
              n222 = in-place-cluster #17("主份控制指令"=w370, "信息帧.数据"=w368) -> (w362:T4)
            }
            n223 = call <vilib>:"Add State(s) to Queue__jki_lib_state_machine.vi"("State(s) in (\"\")"=w361, "State(s) at Back (\"\")"="Request:Write>>1553B_CMD_Beifen") -> ("States Out"=w359:string)  [unwired: 13 in]
          }
          event "主份复位远程终端": Value Change {
            n224 = event-data() -> ()  [unwired: 1 in, 6 out]
            n225 = in-place {
              n226 = in-place-cluster #18(w382) -> ()  [unwired: 1 out]
              n227 = call "1553B_Mode.vi"("模式命令"=u16 8, "RT地址"=u16 16) -> ("1553B指令"=w383:string)  [unwired: 9 in]
              n228 = in-place-cluster #18("信息帧.数据"=w383) -> (w381:T4)
            }
            n229 = call <vilib>:"Add State(s) to Queue__jki_lib_state_machine.vi"("State(s) in (\"\")"=w380, "State(s) at Back (\"\")"="Request:Write>>1553B_CMD_Zhufen") -> ("States Out"=w378:string)  [unwired: 13 in]
          }
          event "备份复位远程终端": Value Change {
            n230 = event-data() -> ()  [unwired: 1 in, 6 out]
            n231 = in-place {
              n232 = in-place-cluster #19(w391) -> ()  [unwired: 1 out]
              n233 = call "1553B_Mode.vi"("模式命令"=u16 8, "RT地址"=u16 16) -> ("1553B指令"=w392:string)  [unwired: 9 in]
              n234 = in-place-cluster #19("信息帧.数据"=w392) -> (w390:T4)
            }
            n235 = call <vilib>:"Add State(s) to Queue__jki_lib_state_machine.vi"("State(s) in (\"\")"=w389, "State(s) at Back (\"\")"="Request:Write>>1553B_CMD_Beifen") -> ("States Out"=w387:string)  [unwired: 13 in]
          }
          event "主份发送器关闭": Value Change {
            n236 = event-data() -> ()  [unwired: 1 in, 6 out]
            n237 = in-place {
              n238 = in-place-cluster #20(w400) -> ()  [unwired: 1 out]
              n239 = call "1553B_Mode.vi"("模式命令"=u16 4, "RT地址"=u16 16) -> ("1553B指令"=w401:string)  [unwired: 9 in]
              n240 = in-place-cluster #20("信息帧.数据"=w401) -> (w399:T4)
            }
            n241 = call <vilib>:"Add State(s) to Queue__jki_lib_state_machine.vi"("State(s) in (\"\")"=w398, "State(s) at Back (\"\")"="Request:Write>>1553B_CMD_Zhufen") -> ("States Out"=w396:string)  [unwired: 13 in]
          }
          event "备份发送器关闭": Value Change {
            n242 = event-data() -> ()  [unwired: 1 in, 6 out]
            n243 = in-place {
              n244 = in-place-cluster #21(w409) -> ()  [unwired: 1 out]
              n245 = call "1553B_Mode.vi"("模式命令"=u16 4, "RT地址"=u16 16) -> ("1553B指令"=w410:string)  [unwired: 9 in]
              n246 = in-place-cluster #21("信息帧.数据"=w410) -> (w408:T4)
            }
            n247 = call <vilib>:"Add State(s) to Queue__jki_lib_state_machine.vi"("State(s) in (\"\")"=w407, "State(s) at Back (\"\")"="Request:Write>>1553B_CMD_Beifen") -> ("States Out"=w405:string)  [unwired: 13 in]
          }
          event "主份取消发送器关闭": Value Change {
            n248 = event-data() -> ()  [unwired: 1 in, 6 out]
            n249 = in-place {
              n250 = in-place-cluster #22(w418) -> ()  [unwired: 1 out]
              n251 = call "1553B_Mode.vi"("模式命令"=u16 5, "RT地址"=u16 16) -> ("1553B指令"=w419:string)  [unwired: 9 in]
              n252 = in-place-cluster #22("信息帧.数据"=w419) -> (w417:T4)
            }
            n253 = call <vilib>:"Add State(s) to Queue__jki_lib_state_machine.vi"("State(s) in (\"\")"=w416, "State(s) at Back (\"\")"="Request:Write>>1553B_CMD_Zhufen") -> ("States Out"=w414:string)  [unwired: 13 in]
          }
          event "备份取消发送器关闭": Value Change {
            n254 = event-data() -> ()  [unwired: 1 in, 6 out]
            n255 = in-place {
              n256 = in-place-cluster #23(w427) -> ()  [unwired: 1 out]
              n257 = call "1553B_Mode.vi"("模式命令"=u16 5, "RT地址"=u16 16) -> ("1553B指令"=w428:string)  [unwired: 9 in]
              n258 = in-place-cluster #23("信息帧.数据"=w428) -> (w426:T4)
            }
            n259 = call <vilib>:"Add State(s) to Queue__jki_lib_state_machine.vi"("State(s) in (\"\")"=w425, "State(s) at Back (\"\")"="Request:Write>>1553B_CMD_Beifen") -> ("States Out"=w423:string)  [unwired: 13 in]
          }
          event "主份发送上一状态字": Value Change {
            n260 = event-data() -> ()  [unwired: 1 in, 6 out]
            n261 = in-place {
              n262 = in-place-cluster #24(w436) -> ()  [unwired: 1 out]
              n263 = call "1553B_Mode.vi"("模式命令"=u16 2, "RT地址"=u16 16) -> ("1553B指令"=w437:string)  [unwired: 9 in]
              n264 = in-place-cluster #24("信息帧.数据"=w437) -> (w435:T4)
            }
            n265 = call <vilib>:"Add State(s) to Queue__jki_lib_state_machine.vi"("State(s) in (\"\")"=w434, "State(s) at Back (\"\")"="Request:Write>>1553B_CMD_Zhufen") -> ("States Out"=w432:string)  [unwired: 13 in]
          }
          event "备份发送上一状态字": Value Change {
            n266 = event-data() -> ()  [unwired: 1 in, 6 out]
            n267 = in-place {
              n268 = in-place-cluster #25(w445) -> ()  [unwired: 1 out]
              n269 = call "1553B_Mode.vi"("模式命令"=u16 2, "RT地址"=u16 16) -> ("1553B指令"=w446:string)  [unwired: 9 in]
              n270 = in-place-cluster #25("信息帧.数据"=w446) -> (w444:T4)
            }
            n271 = call <vilib>:"Add State(s) to Queue__jki_lib_state_machine.vi"("State(s) in (\"\")"=w443, "State(s) at Back (\"\")"="Request:Write>>1553B_CMD_Beifen") -> ("States Out"=w441:string)  [unwired: 13 in]
          }
          event "地检按钮": Value Change {
            n272 = event-data() -> ()  [unwired: 1 in, 6 out]
            n273 = disable-structure shown="启用" {
              disable-tunnel: [w461 _] -> w450
              frame Enabled {
                n274 = local read "陀螺频率"() -> (w458:dbl)
                n275 = local read "陀螺幅值"() -> (w457:dbl)
                n276 = local read "加表幅值"() -> (w459:dbl)
                n277 = call <vilib>:"Sine Waveform.vi"("sampling info"=cluster{"Fs":dbl, "#s":dbl} {"Fs"=100.0, "#s"=100.0}, "amplitude"=w457, "frequency"=w458) -> ("signal out"=w468:waveform(dbl))  [unwired: 7 in, 1 out]
                n278 = local read "加表频率"() -> (w460:dbl)
                n279 = call <vilib>:"Sine Waveform.vi"("sampling info"=cluster{"Fs":dbl, "#s":dbl} {"Fs"=100.0, "#s"=100.0}, "amplitude"=w459, "frequency"=w460) -> ("signal out"=w466:waveform(dbl))  [unwired: 7 in, 1 out]
                n280 = Unbundle By Name(w468) -> ("Y"=w462:dbl[])
                n281 = Unbundle By Name(w466) -> ("Y"=w463:dbl[])
                n282 = Bundle By Name(cluster=cluster{"陀螺":dbl[], "加表":dbl[]} {"陀螺"=[], "加表"=[]} ("输入簇"), "陀螺"=w462, "加表"=w463) -> (w461:cluster{"陀螺":dbl[], "加表":dbl[]})
              }
              frame Disabled {
              }
            }
            n283 = call <vilib>:"Write.vi"("Register name"="DiJian_mode", "Register value"="地检按钮") -> ("Error out"=w449:errorcluster)  [unwired: 11 in, 2 out]
            n284 = call <vilib>:"Write.vi"("Register name"="DiJian_data", "Register value"=w450, "Error in"=w449) -> ()  [unwired: 10 in, 3 out]
          }
          event "陀螺幅值", "陀螺频率", "加表幅值", "加表频率": Value Change {
            n285 = event-data() -> ()  [unwired: 1 in, 6 out]
            n286 = call <vilib>:"Sine Waveform.vi"("sampling info"=cluster{"Fs":dbl, "#s":dbl} {"Fs"=100.0, "#s"=100.0}, "amplitude"="陀螺幅值", "frequency"="陀螺频率") -> ("signal out"=w479:waveform(dbl))  [unwired: 7 in, 1 out]
            n287 = call <vilib>:"Sine Waveform.vi"("sampling info"=cluster{"Fs":dbl, "#s":dbl} {"Fs"=100.0, "#s"=100.0}, "amplitude"="加表幅值", "frequency"="加表频率") -> ("signal out"=w477:waveform(dbl))  [unwired: 7 in, 1 out]
            n288 = Unbundle By Name(w479) -> ("Y"=w473:dbl[])
            n289 = Unbundle By Name(w477) -> ("Y"=w474:dbl[])
            n290 = Bundle By Name(cluster=cluster{"陀螺":dbl[], "加表":dbl[]} {"陀螺"=[], "加表"=[]} ("输入簇"), "陀螺"=w473, "加表"=w474) -> (w482:cluster{"陀螺":dbl[], "加表":dbl[]})
            n291 = call <vilib>:"Write.vi"("Register name"="DiJian_data", "Register value"=w482, "Error in"=w480) -> ("Error out"=w481:errorcluster)  [unwired: 10 in, 2 out]
          }
        }
      }
      frame "---------- Core ----------" {
        # "Do not put any code in this frame.\n(it is a separator no-op)"
        n292 = call <vilib>:"Add State(s) to Queue__jki_lib_state_machine.vi"("State(s) in (\"\")"=w489) -> ("States Out"=w488:string)  [unwired: 14 in]
      }
      frame Default {
        w499 = 42 items=["No error", "Argument error", "Memory is full", "Out of zone", "End of file", "File already open", "Generic file I/O error", "File not found", "File permission error", "Disk is full", "Duplicate path", "Too many files open", "System feature not enabled", "Resource file not found", "Cannot add resource", "Resource not found", "Image not found", "Image memory error", "Pen does not exist", "Config type invalid", "Config token not found", "Config parse error", "Config memory error", "Bad external code format", "Bad external code offset", "External code not present", "Null window", "Destroy window error", "Null menu", "Print aborted", "Bad print record", "Print driver error", "Windows error during printing", "Memory error during printing", "Print dialog error", "Generic print error", "Invalid device refnum", "Device not found", "Device parameter error", "Device unit error", "Cannot open device", "Device call aborted", "Generic error", "Cancelled by user", "Object ID too low", "Object ID too high", "Object not in heap", "Unknown heap", "Unknown object (invalid DefProc)", "Unknown object (DefProc not in table)", "Message out of range", "Invalid (null) method", "Unknown message", "Manager call not supported", "Bad address", "Network operation in progress", "Network operation timed out", "Connection is busy", "Network attribute not supported", "Network error", "Address in use", "System out of memory", "Connection aborted", "Connection refused", "Not connected", "Already connected", "Connection closed", "Initialization error (interapplication manager)", "Bad occurrence", "Wait on unbound occurrence handler", "Occurrence queue overflow", "Datalog type conflict", "Unused", "Unrecognized type (interapplication manager)", "Memory corrupt", "Failed to make temporary DLL", "Old CIN version", "Drag socket not found", "Failed to load drop-object", "Failed to register OLE object", "Failed to release OLE object", "Format specifier type mismatch", "Unknown format specifier", "Too few format specifiers", "Too many format specifiers", "Scan failed", "Newer CIN version", "Error converting to variant", "Runtime menu error", "Password tampered", "Variant attribute not found", "Incompatible variant data type", "Event data is not available", "Event Store is not present", "Occurrence is not found", "Event Queue is not created", "Event info is not available", "Refnum passed is NULL", "Error retrieving Class GUID", "Error retrieving CoClass GUID", "Error retrieving TypeLib GUID.", "Bad built application magic bytes.", "Specific driver is different from the specific driver associated with the Logical Name.", "There is no session opened to the class driver.", "Max Error", "MAX - Error with config objects", "MAX - Error loading configuration", "MAX - Group not supported"]
        # "Current State"
        # "Do not delete, rename, or modify this frame.\n(this is used to capture unhandled states and typos)"
        # "Handle mistyped state name (developer tool)"
        n293 = Format Into String(format string="Software Exception: Unhandled State \"%s\"." ("message"), error in=w495, w490) -> (resulting string=w498:string, error out=w497:errorcluster)  [unwired: 1 in]
        n294 = call <vilib>:"Error Cluster From Error Code.vi"("show call chain? (False)"=TRUE, "error in (no error)"=w497, "error message (\"\")"=w498, "error code (0)"=w499) -> ("error out"=w496:errorcluster)  [unwired: 5 in]
        n295 = call <vilib>:"Add State(s) to Queue__jki_lib_state_machine.vi"("State(s) in (\"\")"=w494) -> ("States Out"=w493:string)  [unwired: 14 in]
      }
      frame "Initialize Core Data" {
        # "Do not delete, rename, or modify this frame.\n(this is used to determine panel behavior on exit)"
        # "originally closed?"
        # "exe?"
        # "If panel starts closed or is an EXE, then close it when we exit"
        n296 = property class="VI"() -> ("Front Panel.Open"=w508:bool)  [unwired: 2 in, 2 out]
        n297 = property class="App"() -> ("App.Kind"=w507:T2)  [unwired: 2 in, 2 out]
        n298 = control-ref of="Current VI Reference"() -> (w501:refnum<vi>)
        n299 = Not(x=w508) -> (.not. x?=w505:bool)
        n300 = Equal?(x=w507, y=T2."Run Time System" ("Application:Kind")) -> (x = y?=w504:bool)
        n301 = Or(x=w505, y=w504) -> (x .or. y?=w502:bool)
        n302 = Bundle By Name(cluster=w503, "Core.Current VI Reference"=w501, "Core.Close Panel on Exit?"=w502) -> (w510:T4)
        n303 = call <vilib>:"Add State(s) to Queue__jki_lib_state_machine.vi"("State(s) in (\"\")"=w512) -> ("States Out"=w511:string)  [unwired: 14 in]
      }
      frame "Error Handler" {
        # "Unhandled Error -- Display it"
        # "Handle any errors here.\nYou can also output any states to clean-up after errors occur"
        # "Clear error"
        n304 = call <vilib>:"General Error Handler.vi"("error in (no error)"=w514) -> ()  [unwired: 10 in, 5 out]
        n305 = call <vilib>:"Add State(s) to Queue__jki_lib_state_machine.vi"("State(s) in Front (\"\")"="/* Post Error States", "State(s) in (\"\")"=w518) -> ("States Out"=w517:string)  [unwired: 13 in]
      }
      frame "Exit" {
        n306 = call <vilib>:"Add State(s) to Queue__jki_lib_state_machine.vi"("State(s) in (\"\")"=w523) -> ("States Out"=w522:string)  [unwired: 14 in]
      }
      frame "---------- Data ----------" {
        # "Do not put any code in this frame.\n(It is a separator no-op. You can make a copy of this frame to create a new Data frame)"
        n307 = call <vilib>:"Add State(s) to Queue__jki_lib_state_machine.vi"("State(s) in (\"\")"=w527) -> ("States Out"=w526:string)  [unwired: 14 in]
      }
      frame "Data: Initialize" {
        w528 = u16 0  # 备份控制指令
        w529 = u16 0  # 主份控制指令
        w531 = T5 {" 数据帧名称"="", " 数据"="", "备用操作符"=TRUE, "起始地址"=0, "读写标志"=0, "长度"=0}  # 信息帧
        w532 = T6 {"Current VI Reference"=refnum, "Close Panel on Exit?"=FALSE}  # Core
        n308 = Bundle("Core"=w532, "传递队列输入"=w530, "信息帧"=w531, "主份控制指令"=w529, "备份控制指令"=w528) -> (w534:T4)  [unwired: 1 in]
        n309 = call <vilib>:"Add State(s) to Queue__jki_lib_state_machine.vi"("State(s) in (\"\")"=w536) -> ("States Out"=w535:string)  [unwired: 14 in]
      }
      frame "Data: Cleanup" {
        # "Cleanup any data and references, here.\n(this is called automatically, by the Macro: Exit)"
        n310 = Unbundle By Name(w537) -> ("Core.Current VI Reference"=w540:refnum<vi>)
        n311 = Close Reference(reference=w540, error in (no error)=w539) -> (error out=w538:errorcluster)
        n312 = call <vilib>:"Add State(s) to Queue__jki_lib_state_machine.vi"("State(s) in (\"\")"=w542) -> ("States Out"=w541:string)  [unwired: 14 in]
      }
      frame "---------- UI ----------" {
        # "Do not put any code in this frame.\n(It is a separator no-op. You can make a copy of this frame to create a new UI frame)"
        n313 = call <vilib>:"Add State(s) to Queue__jki_lib_state_machine.vi"("State(s) in (\"\")"=w546) -> ("States Out"=w545:string)  [unwired: 14 in]
      }
      frame "UI: Initialize" {
        # "Initialize the User Interface, here.\n(this is called automatically, by the Macro: Init)"
        n314 = call <vilib>:"Add State(s) to Queue__jki_lib_state_machine.vi"("State(s) in (\"\")"=w550) -> ("States Out"=w549:string)  [unwired: 14 in]
      }
      frame "UI: Cursor Set" {
        # "Argument"
        # "Set and Unset Cursor Busy.\n(Usage: \"UI: Cursor Set >> Busy|Idle\")"
        n315 = case shown="\"Idle\", 默认" w551 {
          tunnel: w553 -> [w558 w560]
          tunnel: [w557 w559] -> w552
          frame "Idle", Default {
            n316 = call <vilib>:"Unset Busy.vi"("error in (no error)"=w558) -> ("error out"=w557:errorcluster)  [unwired: 10 in]
          }
          frame "Busy" {
            n317 = call <vilib>:"Set Busy.vi"("error in (no error)"=w560) -> ("error out"=w559:errorcluster)  [unwired: 9 in, 1 out]
          }
        }
        n318 = call <vilib>:"Add State(s) to Queue__jki_lib_state_machine.vi"("State(s) in (\"\")"=w556) -> ("States Out"=w555:string)  [unwired: 14 in]
      }
      frame "UI: Front Panel State" {
        # "Set Front Panel Open or Closed\n(Usage: \"UI: Front Panel State >> Open|Close\")"
        n319 = disable-structure shown="启用" {
          disable-tunnel: w564 -> [w571 w594]
          disable-tunnel: [w570 w594] -> w563
          disable-tunnel: w562 -> [w569 _]
          disable-tunnel: w561 -> [w567 _]
          frame Disabled {
            # "Argument"
            n320 = Unbundle By Name(w569) -> ("Core.Current VI Reference"=w568:refnum<vi>)
            n321 = case shown="\"Open\", 默认" w567 {
              tunnel: w571 -> [w575 w588]
              tunnel: [w577 w589] -> w570
              tunnel: w568 -> [w576 w586]
              frame "Open", Default {
                n322 = property class="VI"(reference=w576, error in=w575) -> (reference out=w573:refnum<vi>, error out=w574:errorcluster, "Front Panel.Open"=w572:bool)
                n323 = case shown="假" w572 {
                  tunnel: [w580 w583] -> w577
                  tunnel: w574 -> [w579 w583]
                  tunnel: w573 -> [w578 _]
                  frame False {
                    n324 = invoke class="VI" method="FP.Open"(reference=w578, error in=w579, "Activate"=TRUE, "State"=T3."Standard") -> (error out=w580:errorcluster)  [unwired: 1 in, 4 out]
                  }
                  frame True {
                  }
                }
              }
              frame "Close" {
                n325 = property class="VI"(reference=w586, error in=w588) -> (reference out=w585:refnum<vi>, error out=w587:errorcluster, "Front Panel.Open"=w584:bool)
                n326 = case shown="真" w584 {
                  tunnel: [w590 w593] -> w589
                  tunnel: w587 -> [w590 w592]
                  tunnel: w585 -> [_ w591]
                  frame False {
                  }
                  frame True {
                    n327 = invoke class="VI" method="FP.Close"(reference=w591, error in=w592) -> (error out=w593:errorcluster)  [unwired: 1 in, 2 out]
                  }
                }
              }
            }
          }
          frame Enabled {
          }
        }
        n328 = call <vilib>:"Add State(s) to Queue__jki_lib_state_machine.vi"("State(s) in (\"\")"=w566) -> ("States Out"=w565:string)  [unwired: 14 in]
      }
      frame "---------- Macro ----------" {
        # "Do not put any code in this frame.\n(It is a separator no-op. You can make a copy of this frame to create a new Macro frame)"
        n329 = call <vilib>:"Add State(s) to Queue__jki_lib_state_machine.vi"("State(s) in (\"\")"=w598) -> ("States Out"=w597:string)  [unwired: 14 in]
      }
      frame "Macro: Initialize" {
        w599 = "Data: Initialize\nInitialize Core Data\nUI: Initialize\nUI: Front Panel State >> Open"  # Data: Initialize Initialize Core Data UI: Initialize UI: Front Panel State >> Open
        # "Initialization Macro\n(This is called once, when the VI starts)"
        n330 = call <vilib>:"Add State(s) to Queue__jki_lib_state_machine.vi"("State(s) in Front (\"\")"=w599, "State(s) in (\"\")"=w603) -> ("States Out"=w602:string)  [unwired: 13 in]
      }
      frame "Macro: Exit" {
        # "Exit Macro\n(This is called once, when the VI exits)"
        n331 = Unbundle By Name(w610) -> ("Core.Close Panel on Exit?"=w609:bool)
        n332 = Select(t="UI: Front Panel State >> Close", s=w609, f="") -> (s? t:f=w606:string)
        n333 = call <vilib>:"Add State(s) to Queue__jki_lib_state_machine.vi"("State(s) in (\"\")"=w606, "State(s) at Back (\"\")"="Data: Cleanup\nExit") -> ("States Out"=w604:string)  [unwired: 13 in]
        n334 = call <vilib>:"Add State(s) to Queue__jki_lib_state_machine.vi"("State(s) in Front (\"\")"=w604, "State(s) in (\"\")"=w613) -> ("States Out"=w612:string)  [unwired: 13 in]
      }
      frame "----------Request----------" {
        # "Template Separator\n(You can make a copy of, or modify, this frame)"
        n335 = call <vilib>:"Add State(s) to Queue__jki_lib_state_machine.vi"("State(s) in (\"\")"=w617) -> ("States Out"=w616:string)  [unwired: 14 in]
      }
      frame "Request:Write" {
        n336 = in-place {
          in-place-border: w621 -> [w627]
          in-place-border: [w626] -> w620
          in-place-border: w618 -> [w625]
          n337 = in-place-cluster #26(w622) -> ("传递队列输入"=w631:refnum<queue>, "信息帧"=w630:T5)
          n338 = in-place {
            in-place-border: w625 -> [w632]
            n339 = in-place-cluster #27(w630) -> ("数据"=w637:string)  [unwired: 5 out]
            n340 = in-place-cluster #27("数据帧名称"=w632, "数据"=w637, "备用操作符"=TRUE, "起始地址"=0, "读写标志"=1, "长度"=0) -> (w629:T5)
          }
          n341 = Enqueue Element(queue=w631, element=w629, error in (no error)=w627) -> (queue out=w628:refnum<queue>, error out=w626:errorcluster)  [unwired: 1 in, 1 out]
          n342 = in-place-cluster #26("传递队列输入"=w628, "信息帧"=w629) -> (w619:T4)
        }
        n343 = call <vilib>:"Add State(s) to Queue__jki_lib_state_machine.vi"("State(s) in (\"\")"=w624) -> ("States Out"=w623:string)  [unwired: 14 in]
      }
      frame "Request:OPEN1553B" {
        n344 = in-place {
          in-place-border: w641 -> [w648]
          in-place-border: [w647] -> w640
          in-place-border: w638 -> [w645]
          n345 = in-place-cluster #28(w642) -> ("传递队列输入"=w651:refnum<queue>, "信息帧"=w646:T5)
          n346 = in-place {
            in-place-border: w645 -> [w652]
            n347 = in-place-cluster #29(w646) -> ()  [unwired: 6 out]
            n348 = in-place-cluster #29("数据帧名称"=w652, "数据"="$B\n", "备用操作符"=TRUE, "起始地址"=0, "读写标志"=1, "长度"=0) -> (w650:T5)
          }
          n349 = Enqueue Element(queue=w651, element=w650, error in (no error)=w648) -> (queue out=w649:refnum<queue>, error out=w647:errorcluster)  [unwired: 1 in, 1 out]
          n350 = in-place-cluster #28("传递队列输入"=w649, "信息帧"=w646) -> (w639:T4)
        }
        n351 = call <vilib>:"Add State(s) to Queue__jki_lib_state_machine.vi"("State(s) in (\"\")"=w644) -> ("States Out"=w643:string)  [unwired: 14 in]
      }
      frame "Request:Close1553B" {
        n352 = in-place {
          in-place-border: w660 -> [w669]
          in-place-border: [w668] -> w659
          n353 = in-place-cluster #30(w661) -> ("传递队列输入"=w671:refnum<queue>, "信息帧"=w665:T5)
          n354 = in-place {
            n355 = in-place-cluster #31(w665) -> ()  [unwired: 6 out]
            n356 = in-place-cluster #31("数据帧名称"="1553B_CMD", "数据"="$", "备用操作符"=TRUE, "起始地址"=0, "读写标志"=1, "长度"=0) -> (w670:T5)
          }
          n357 = in-place {
            n358 = in-place-cluster #32(w665) -> ()  [unwired: 6 out]
            n359 = in-place-cluster #32("数据帧名称"="1553B_CMD", "数据"="$Z\n", "备用操作符"=TRUE, "起始地址"=0, "读写标志"=1, "长度"=0) -> (w666:T5)
          }
          n360 = Enqueue Element(queue=w671, element=w670, error in (no error)=w669) -> (queue out=w667:refnum<queue>, error out=w668:errorcluster)  [unwired: 1 in, 1 out]
          n361 = Enqueue Element(queue=w667, element=w666) -> (queue out=w664:refnum<queue>)  [unwired: 2 in, 2 out]
          n362 = in-place-cluster #30("传递队列输入"=w664, "信息帧"=w665) -> (w658:T4)
        }
        n363 = call <vilib>:"Add State(s) to Queue__jki_lib_state_machine.vi"("State(s) in (\"\")"=w663) -> ("States Out"=w662:string)  [unwired: 14 in]
      }
      frame "Request:Read" {
        n364 = in-place {
          in-place-border: w686 -> [w691]
          in-place-border: [w690] -> w685
          n365 = in-place-cluster #33(w687) -> ("传递队列输入"=w695:refnum<queue>, "信息帧"=w694:T5)
          n366 = in-place {
            n367 = in-place-cluster #34(w694) -> ("数据"=w700:string)  [unwired: 5 out]
            n368 = in-place-cluster #34("数据帧名称"="GNSS1", "数据"=w700, "备用操作符"=TRUE, "起始地址"=0, "读写标志"=0, "长度"=0) -> (w693:T5)
          }
          n369 = Enqueue Element(queue=w695, element=w693, error in (no error)=w691) -> (queue out=w692:refnum<queue>, error out=w690:errorcluster)  [unwired: 1 in, 1 out]
          n370 = in-place-cluster #33("传递队列输入"=w692, "信息帧"=w693) -> (w684:T4)
        }
        n371 = call <vilib>:"Add State(s) to Queue__jki_lib_state_machine.vi"("State(s) in (\"\")"=w689) -> ("States Out"=w688:string)  [unwired: 14 in]
      }
      frame "----------Usr----------" {
        # "Template Separator\n(You can make a copy of, or modify, this frame)"
        n372 = call <vilib>:"Add State(s) to Queue__jki_lib_state_machine.vi"("State(s) in (\"\")"=w705) -> ("States Out"=w704:string)  [unwired: 14 in]
      }
      frame "Usr:Exit" {
        n373 = call <vilib>:"Add State(s) to Queue__jki_lib_state_machine.vi"("State(s) in Front (\"\")"="Macro: Exit", "State(s) in (\"\")"=w710) -> ("States Out"=w709:string)  [unwired: 13 in]
      }
      frame "Usr:Frame-init" {
        n374 = in-place {
          n375 = in-place-cluster #35(w712) -> ()  [unwired: 1 out]
          n376 = Initialize Array(u8 0 ("元素"), 218 ("维数大小")) -> (w719:u8[])
          n377 = Replace Array Subset(array=w719, new element=u8[] [170, 85, 218, 0], index=0 ("索引")) -> (w716:u8[])
          n378 = Byte Array To String(unsigned byte array=w716) -> (string=w722:string)
          n379 = in-place-cluster #35("信息帧.数据"=w722) -> (w711:T4)
        }
        n380 = call <vilib>:"Add State(s) to Queue__jki_lib_state_machine.vi"("State(s) in (\"\")"=w715) -> ("States Out"=w714:string)  [unwired: 14 in]
      }
      frame "Usr:Frame-set" {
        n381 = disable-structure shown="禁用" {
          disable-tunnel: ["Request:Write" ("State(s) in Front (\"\")") _] -> w724
          frame Disabled {
          }
          frame Enabled {
          }
        }
        n382 = call <vilib>:"Add State(s) to Queue__jki_lib_state_machine.vi"("State(s) in (\"\")"=w727, "State(s) at Back (\"\")"=w724) -> ("States Out"=w726:string)  [unwired: 13 in]
      }
    }
  }
  n383 = while {
    tunnel: "notifier" -> [w738]
    stop <- w737 stop-if-true
    n384 = call "stop_message_vmc.vi"("notifier"=w738) -> ("Exit？"=w737:bool)  [unwired: 9 in, 1 out]
    n385 = call <vilib>:"Read.vi"("Timeout"=1, "Register name"="1553BBeiFenRecv") -> ("Register value"=w732:variant, "Register value read?"=w731:bool)  [unwired: 10 in, 2 out]
    n386 = call <vilib>:"Read.vi"("Timeout"=1, "Register name"="1553BZhuFenRecv") -> ("Register value"=w733:variant, "Register value read?"=w734:bool)  [unwired: 10 in, 2 out]
    n387 = case shown="真" w731 {
      tunnel: w732 -> [_ w745]
      frame False {
      }
      frame True {
        n388 = call-poly <vilib>:"Convert.vi"("Register value in"=w745) -> ("Register value out"=w744:string)  [unwired: 13 in, 1 out]
        n389 = String To Byte Array(string=w744) -> (unsigned byte array=w743:u8[])
        n390 = Array Subset(array=w743, index=0 ("索引"), length=42 ("长度")) -> (w739:u8[])
        n391 = case shown="真" TRUE {
          tunnel: w739 -> [_ w769]
          frame False {
          }
          frame True {
            n392 = call "1553B_帧解析.vi"("数组"=w769) -> ("帧数据"=w768:T7)  [unwired: 10 in]
            n393 = Unbundle By Name(w768) -> ("G1陀螺自检状态"=w766:u8, "G2陀螺自检状态"=w762:u8, "G3陀螺自检状态"=w763:u8, "A1自检状态"=w757:u8, "A2自检状态"=w755:u8, "A3自检状态"=w756:u8, "温控自检字"=w748:u8)  [unwired: 19 out]
            n394 = call "陀螺状态自检.vi"("G123"="G3", "陀螺自检状态字"=w763) -> ("连接的字符串"=w758:string)  [unwired: 9 in]
            n395 = call "陀螺状态自检.vi"("G123"="G2", "陀螺自检状态字"=w762) -> ("连接的字符串"=w759:string)  [unwired: 9 in]
            n396 = call "陀螺状态自检.vi"("G123"="G1", "陀螺自检状态字"=w766) -> ("连接的字符串"=w764:string)  [unwired: 9 in]
            n397 = call "加计状态自检.vi"("G123"="A3", "加速度计自检状态字"=w756) -> ("连接的字符串"=w749:string)  [unwired: 9 in]
            n398 = call "加计状态自检.vi"("G123"="A2", "加速度计自检状态字"=w755) -> ("连接的字符串"=w750:string)  [unwired: 9 in]
            n399 = call "温控状态.vi"("温控状态字"=w748) -> ("连接的字符串"=w747:string)  [unwired: 10 in]
            n400 = call "加计状态自检.vi"("G123"="A1", "加速度计自检状态字"=w757) -> ("连接的字符串"=w751:string)  [unwired: 9 in]
            n401 = Concatenate Strings("陀螺就、加计自检状态\n\n" ("字符串"), w764, w759, w758, w751, w750, w749, w747) -> (→"备份自检状态及船舱标志":string)
          }
        }
      }
    }
    n402 = case shown="真" w734 {
      tunnel: w733 -> [_ w776]
      frame False {
      }
      frame True {
        n403 = call-poly <vilib>:"Convert.vi"("Register value in"=w776) -> ("Register value out"=w775:string)  [unwired: 13 in, 1 out]
        n404 = String To Byte Array(string=w775) -> (unsigned byte array=w774:u8[])
        n405 = Array Subset(array=w774, index=0 ("索引"), length=42 ("长度")) -> (w770:u8[])
        n406 = case shown="真" TRUE {
          tunnel: w770 -> [_ w800]
          frame False {
          }
          frame True {
            n407 = call "1553B_帧解析.vi"("数组"=w800) -> ("帧数据"=w799:T7)  [unwired: 10 in]
            n408 = Unbundle By Name(w799) -> ("G1陀螺自检状态"=w797:u8, "G2陀螺自检状态"=w793:u8, "G3陀螺自检状态"=w794:u8, "A1自检状态"=w788:u8, "A2自检状态"=w786:u8, "A3自检状态"=w787:u8, "温控自检字"=w779:u8)  [unwired: 19 out]
            n409 = call "陀螺状态自检.vi"("G123"="G3", "陀螺自检状态字"=w794) -> ("连接的字符串"=w789:string)  [unwired: 9 in]
            n410 = call "陀螺状态自检.vi"("G123"="G2", "陀螺自检状态字"=w793) -> ("连接的字符串"=w790:string)  [unwired: 9 in]
            n411 = call "陀螺状态自检.vi"("G123"="G1", "陀螺自检状态字"=w797) -> ("连接的字符串"=w795:string)  [unwired: 9 in]
            n412 = call "加计状态自检.vi"("G123"="A3", "加速度计自检状态字"=w787) -> ("连接的字符串"=w780:string)  [unwired: 9 in]
            n413 = call "加计状态自检.vi"("G123"="A2", "加速度计自检状态字"=w786) -> ("连接的字符串"=w781:string)  [unwired: 9 in]
            n414 = call "温控状态.vi"("温控状态字"=w779) -> ("连接的字符串"=w778:string)  [unwired: 10 in]
            n415 = call "加计状态自检.vi"("G123"="A1", "加速度计自检状态字"=w788) -> ("连接的字符串"=w782:string)  [unwired: 9 in]
            n416 = Concatenate Strings("陀螺就、加计自检状态\n\n" ("字符串"), w795, w790, w789, w782, w781, w780, w778) -> (→"主份自检状态及船舱标志":string)
          }
        }
      }
    }
  }
